vi "r3_Pick&Place_module_sensor_glueDespRev.vi"() -> ()   [LabVIEW 2016]
uses:
  Classes/Controllers/I-O/Copy of NI-DAQ Folder/NI-DAQ.lvclass
  D:/INTT/V1/Classes/Controllers/I-O/Copy of I-O Folder/I-O.lvclass
  Classes/Controllers/Dispenser/Copy of Ultimus V2 Folder/Ultimus V2.lvclass
  <vilib>/Analysis/coordinate.llb/2D Cartesian Coordinate Rotation (Scalar).vi
  <vilib>/Utility/file.llb/Read Delimited Spreadsheet (DBL).vi
  <vilib>/Utility/file.llb/Write Delimited Spreadsheet (DBL).vi
  Classes/Controllers/Motion/Copy of Motion Folder/Motion.lvclass
  Classes/Controllers/Camera/Copy of Controller Folder/Controller.lvclass
  <vilib>/Analysis/NI_AALPro.lvlib
  Classes/Controllers/I-O/Copy of I-O Folder/I-O.lvclass
panel:
  in  "sensor pad offset":dbl[][](array[numeric])=[[0.01279, -0.02707, 0.0, 0.0], [0.02738, -0.01377, 0.0, 0.0]]
  out "Sample on HDI aspect to drawing":dbl[][](array[numeric]) format="%#_8g"
  in  "HDI sensor pad positions":dbl[][](array[numeric]) format="%#_12g"
  in  "Values":bool[](array[boolean])=[FALSE, FALSE]
  out "vacuum on?":bool[](array[boolean])
  out "Array 2":dbl[][](array[numeric])
  out "Measured PickupTool position":dbl[][](array[numeric])
  in  "sampel vacuum":i32[](array[numeric])=[15, 19]
  in  "VacChannel for sample":i32=1
  in  "TrayVaccum":bool
  in  "check height? 2":bool
  in  "check height?":bool
  out "Needle parking position":dbl[](array[numeric])
  out "GlueBox":dbl[][](array[numeric])
  out "appended array":dbl[][](array[numeric])
  in  "chip placement height compensation":dbl=-0.47 format="%#_13g"
  out "Sample on HDI":dbl[][](array[numeric]) format="%#_8g"
  in  "Sensor A/B":bool
  out "Gantry current position":dbl[](array[numeric])
  in  "READ Position":bool
  in  "Needle Height Compenstation\n(glue gap)":dbl=0.34
  in  "Needle Alignment":bool
  in  "Parking position":dbl[](array[numeric])=[500.0, 625.0, 0.0, 0.01]
  in  "GOTO":bool
  in  "Default Pickup Tool Position":dbl[][](array[numeric])=[[132.189, 676.043, 47.1693, 0.0326839], [189.108, 526.841, 47.062, 0.0198801]]
  in  "Number of Chips/Sensors \nto be assembled":i32=1
  in  "Default HDI alignment \nmark position":dbl[](array[numeric])=[292.31, 988.829, 78.9737, -0.000591208]
  in  "Default HDI size":dbl[](array[numeric])=[24.3157, 231.332, -0.00999644, -6.1789e-05]
  out "# of tasks excuted":i32
  out "Chips on tray position":dbl[][](array[numeric])
  out "measured HDI size":dbl[](array[numeric])
  in  "Chip tray":dbl[](array[numeric])=[465.031, 710.639, 69.8028, 0.00407755]
  out "Sample position \non HDI":dbl[][](array[numeric]) format="%#_8g"
  in  "Inititalize":bool
  in  "Pick and place":bool
  in  "Deposit Glue":bool
  in  "Measure Pickup Tools":bool
  in  "Measure Samples on tray":bool
  out "default chip and sensor position w.r.t. 1st mark":dbl[][](array[numeric])
  in  "Assembly Type":bool
  in  "Stop":bool
  in  "Measure HDI":bool
  out "Measure HDI top-left":dbl[](array[numeric])
  # "Sensor Tray \nVacuum Channel"
  # "Chips"
  # "Sensor 0.3 -> 200 micron glue thickness\nChips 0.34-> 150 micron glue thickness"
  # "Sensors"
  # "Sensor B short"
  # "Sensors B\n(Short)"
  # "Sensors A\n(Long)"
  # "Chips : -0.47-> 60 micron height gap\n               -0.5 -> 90 micron"
  # "Sensor A long"
  # "ACTIONS"
  # "HDI infomation"
  # "sensor"
  # "chips use channel 0, 2\nsensors use channel 0, 1"
  # "sensor height 69.8471\nchip height 84.693"
  # "Pick and Place"
  # "TYPE A: \nX: 0.01279\nY: -0.02707"
  # "TYPE B: \nX: 0.02738\nY: -0.01377"
  # "type A"
  # "type B"
  # "type A"
  # "type B"
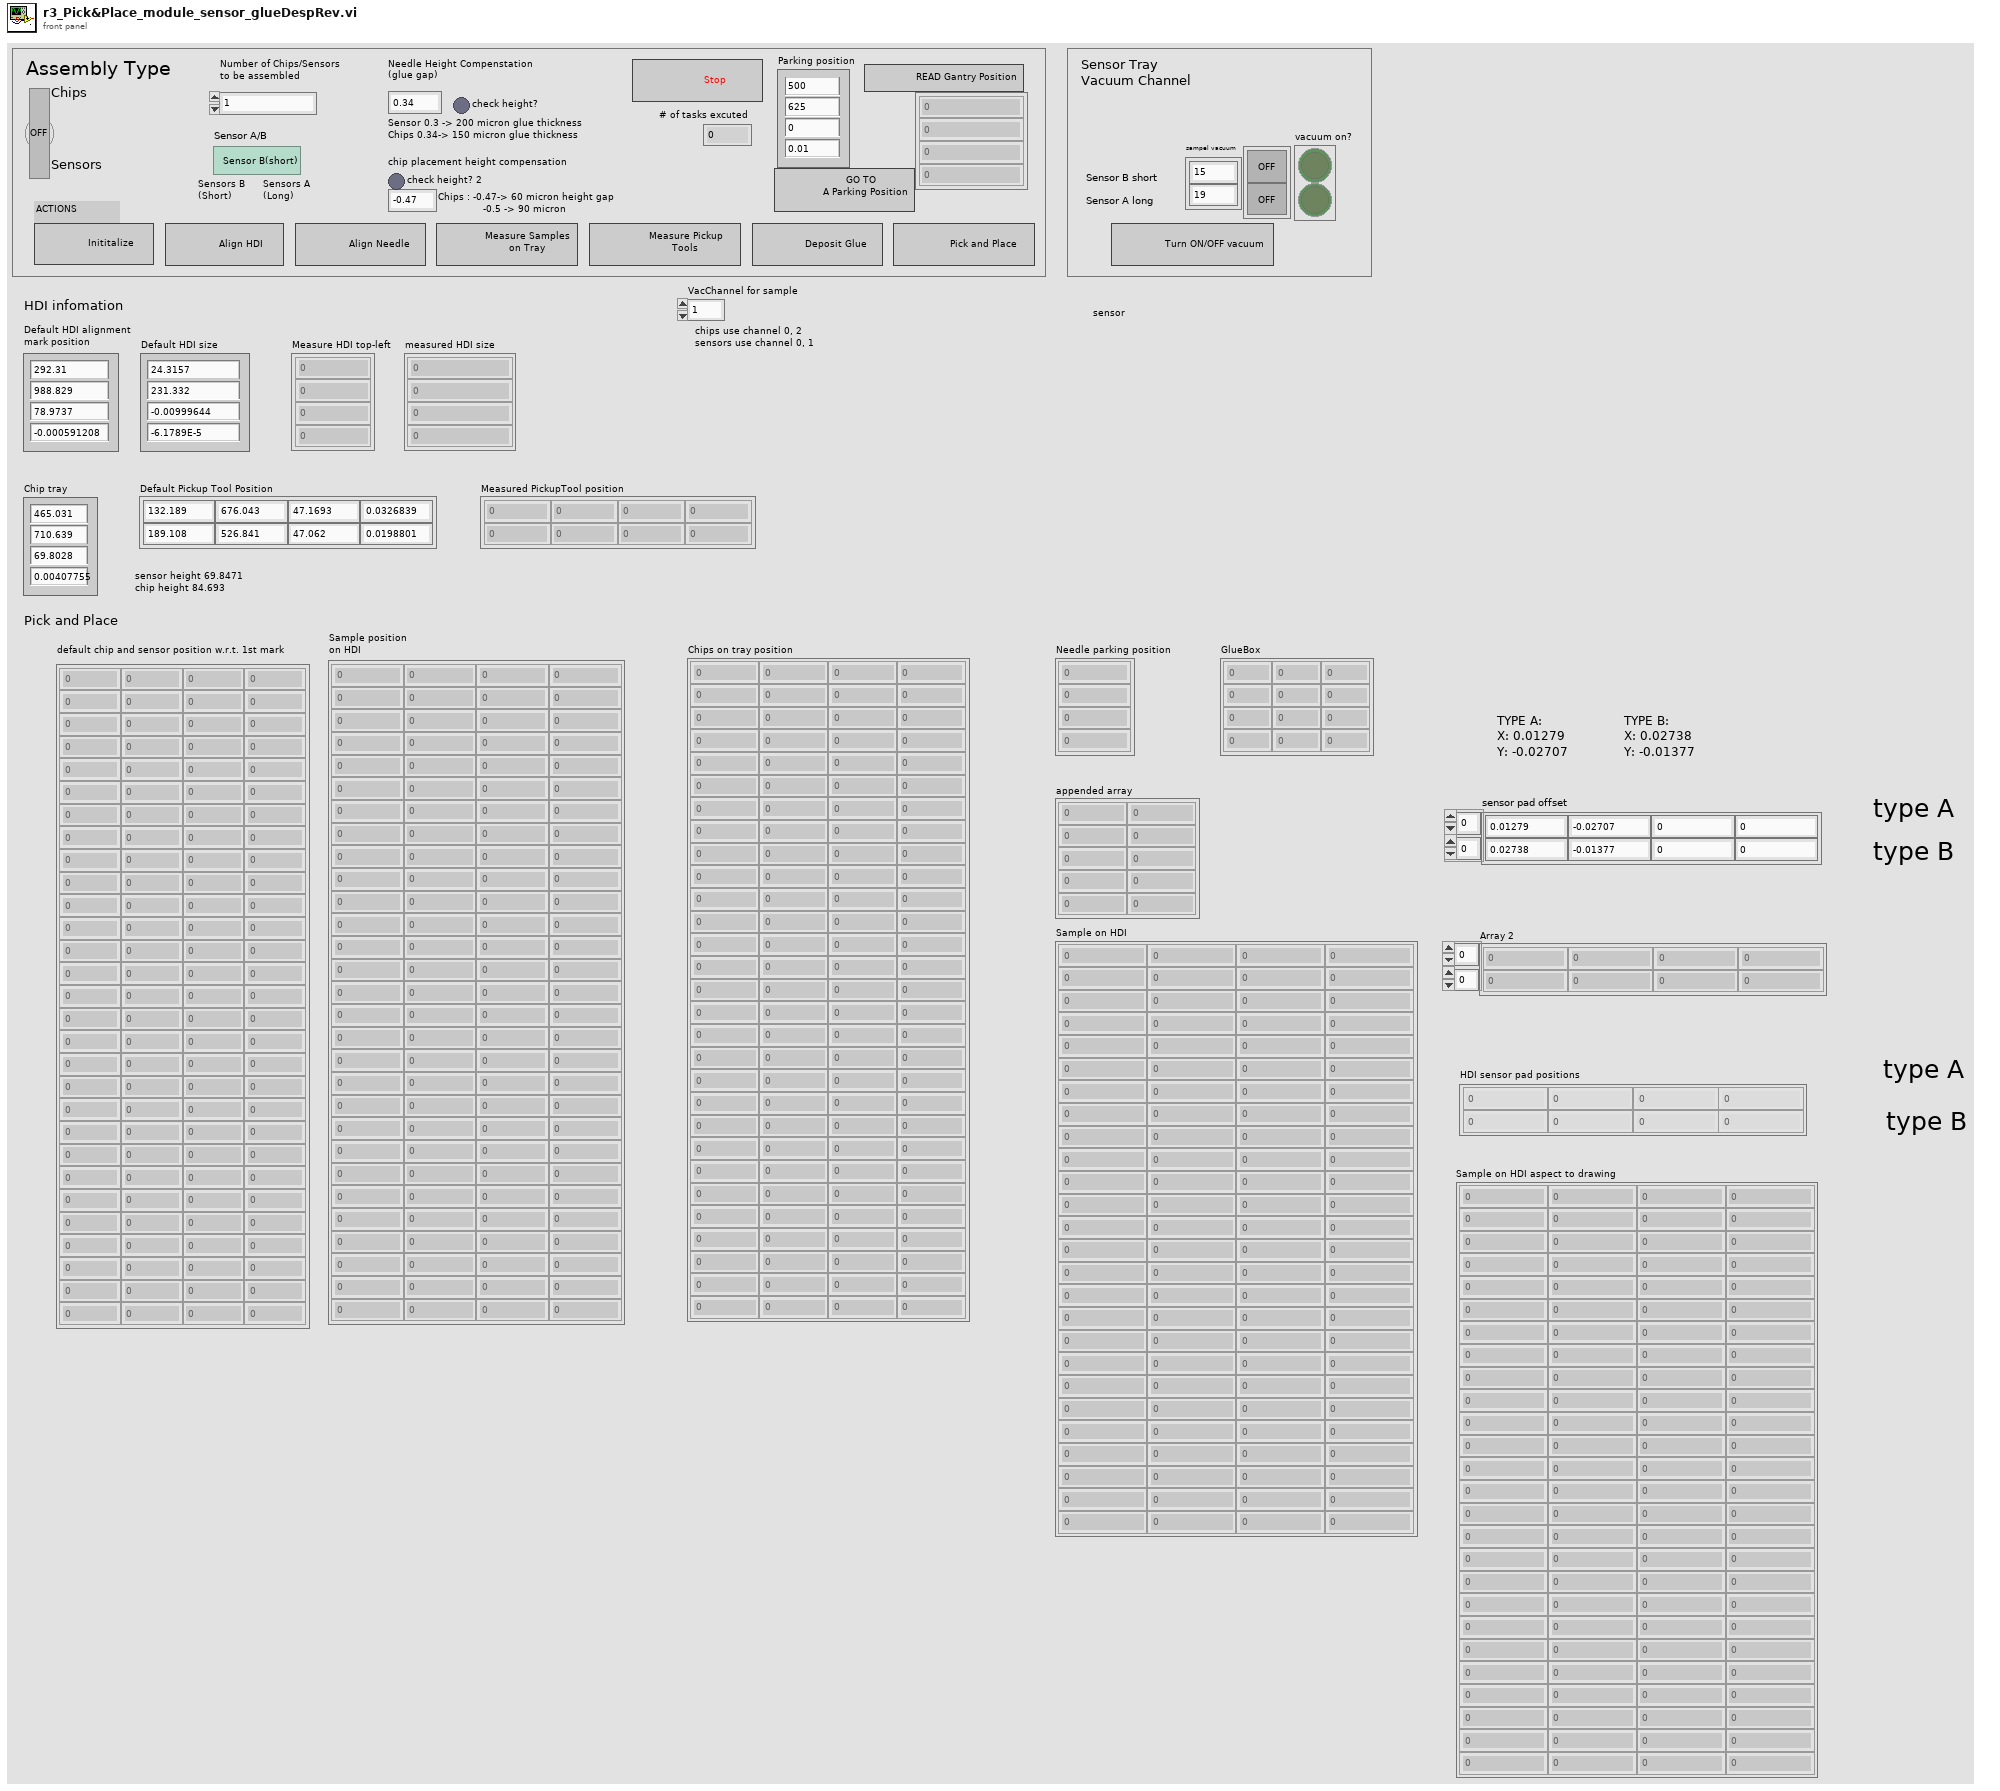
[diagram p1: front panel]
types:
  T1 = typedef "Controller.lvclass/Controllers.ctl" = cluster{"Copy of Motion.lvclass":refnum<class "Motion.lvclass">, "Copy of I-O.lvclass":refnum<class "I-O.lvclass">, "Copy of Dispenser.lvclass":refnum<class "Dispenser.lvclass">}
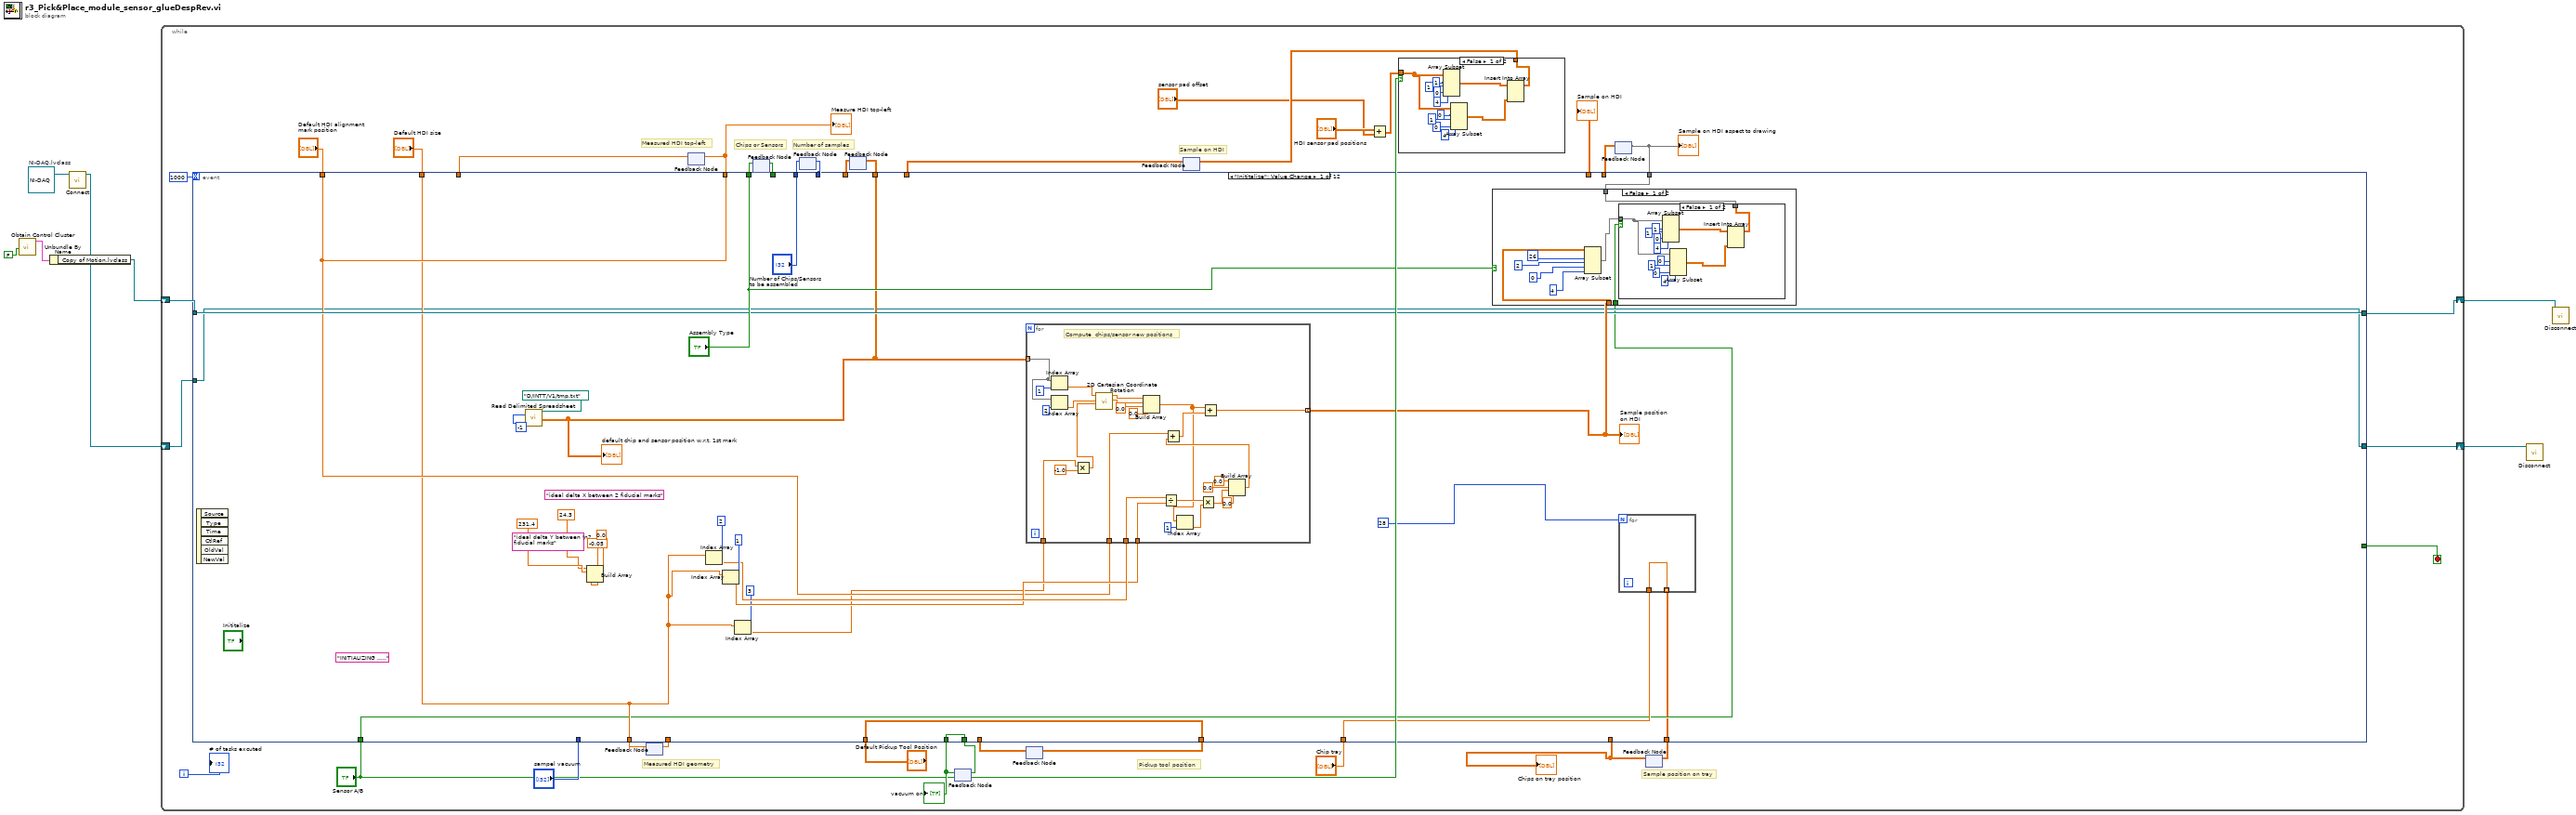
[diagram p0: block diagram]
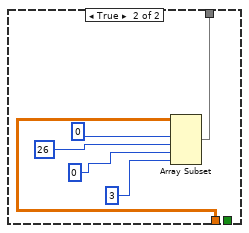
[diagram p4: hidden frame]
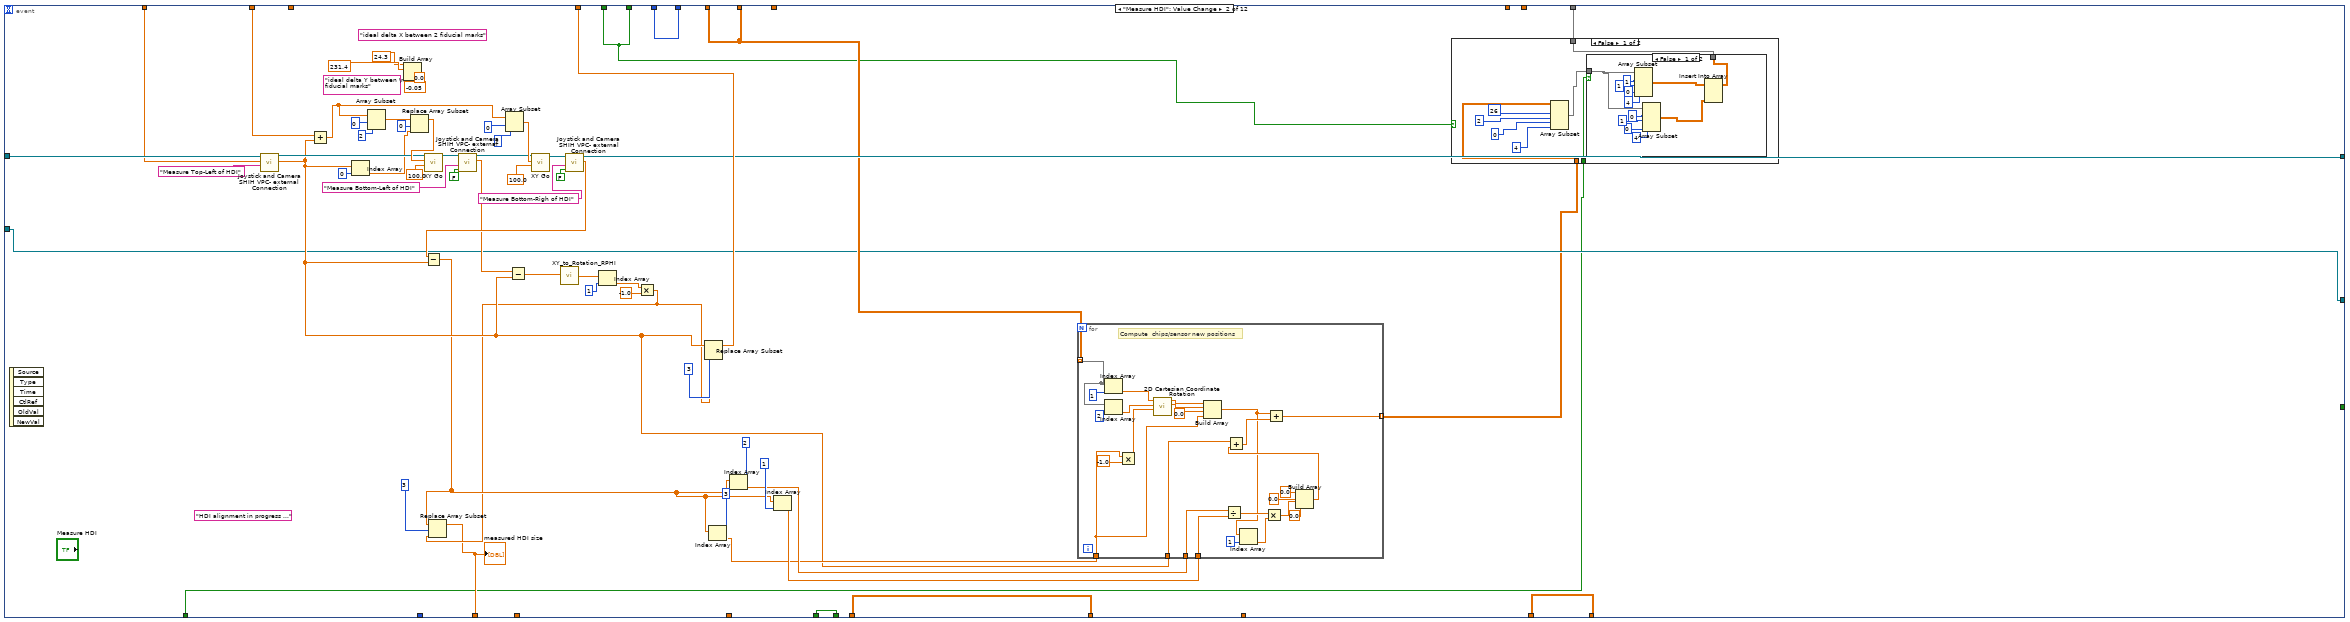
[diagram p5: hidden frame]
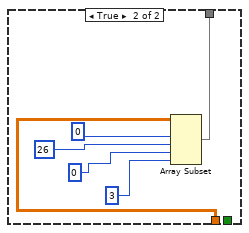
[diagram p7: hidden frame]
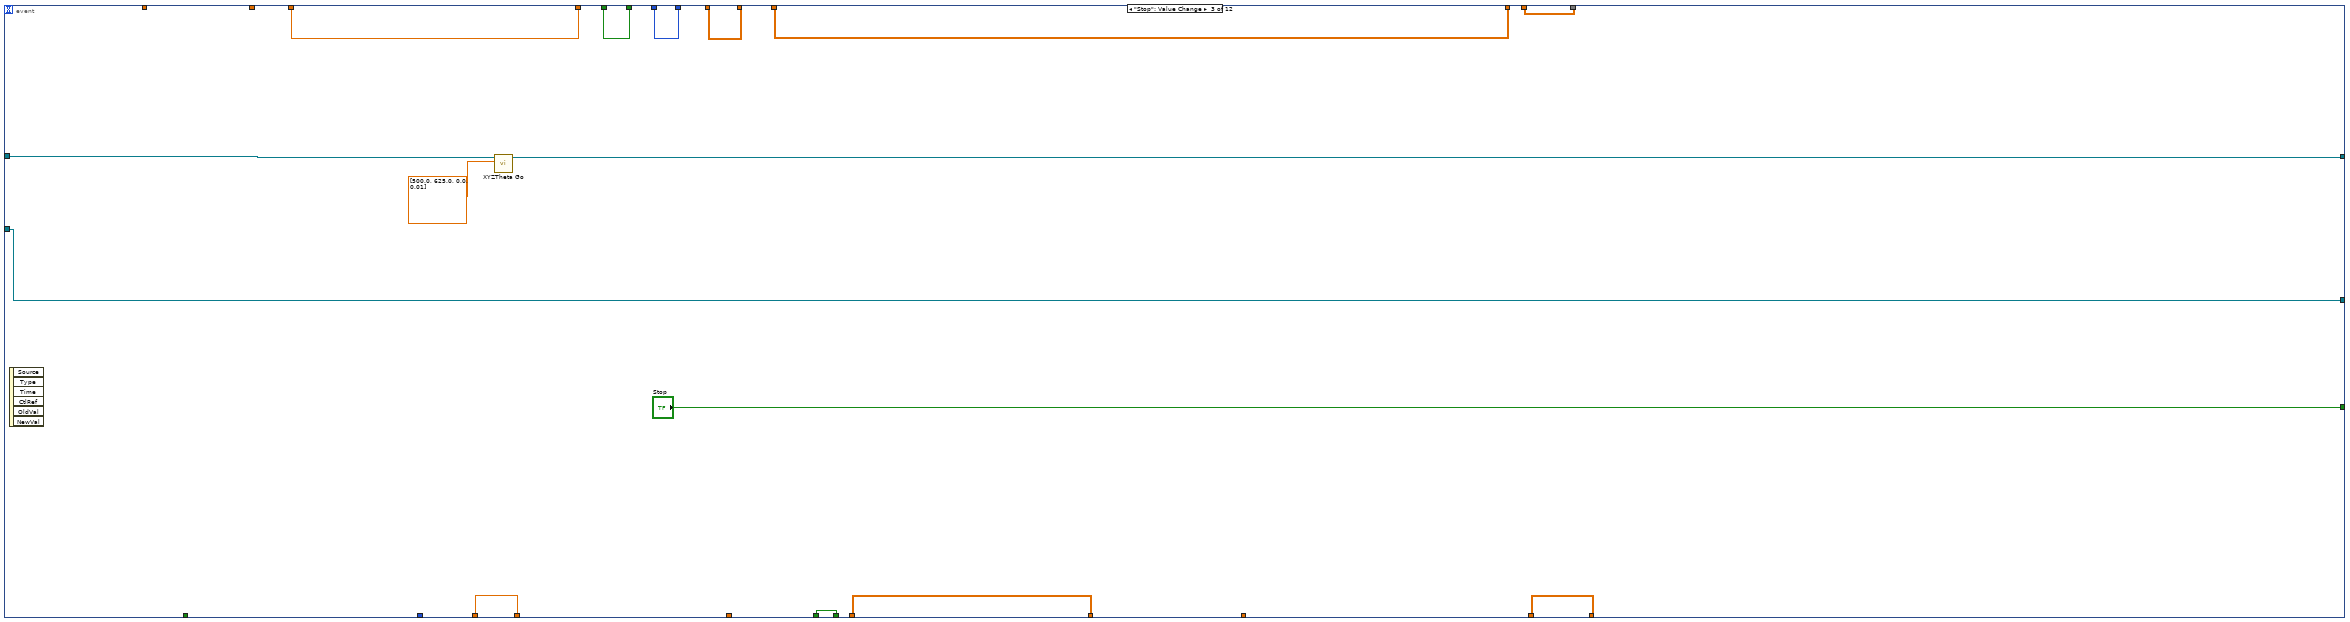
[diagram p8: hidden frame]
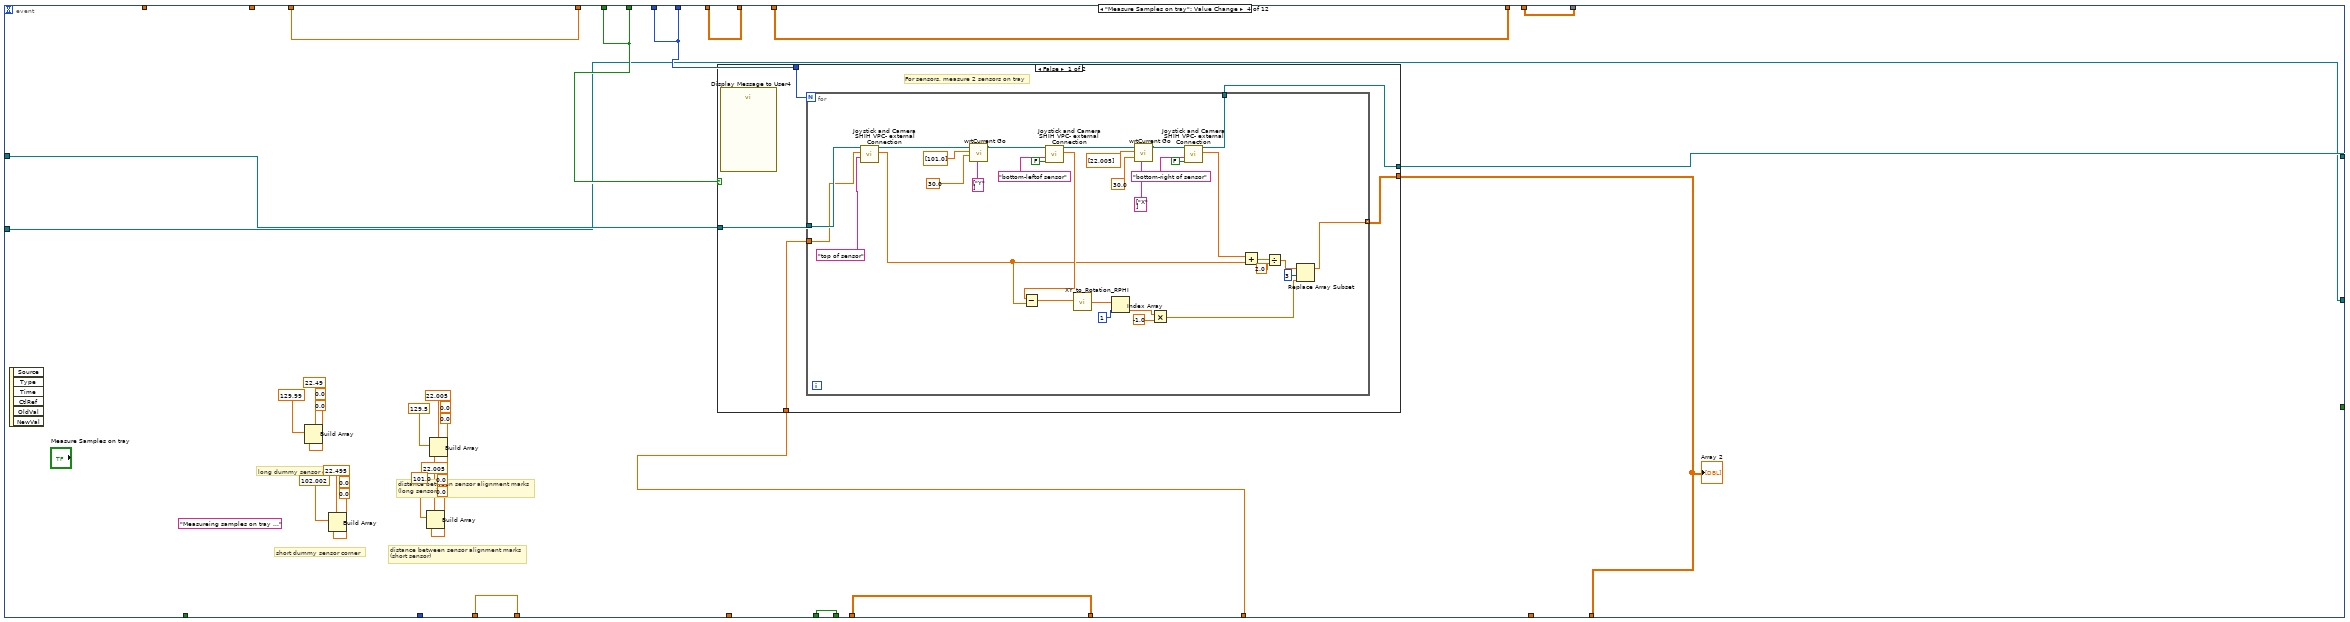
[diagram p9: hidden frame]
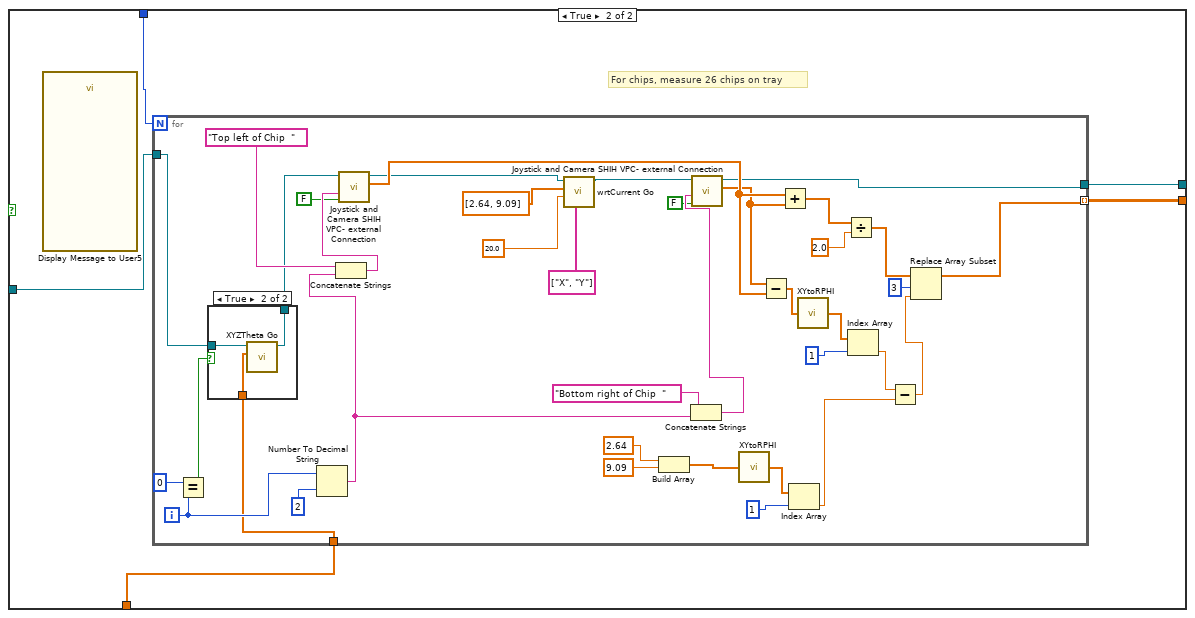
[diagram p10: hidden frame]
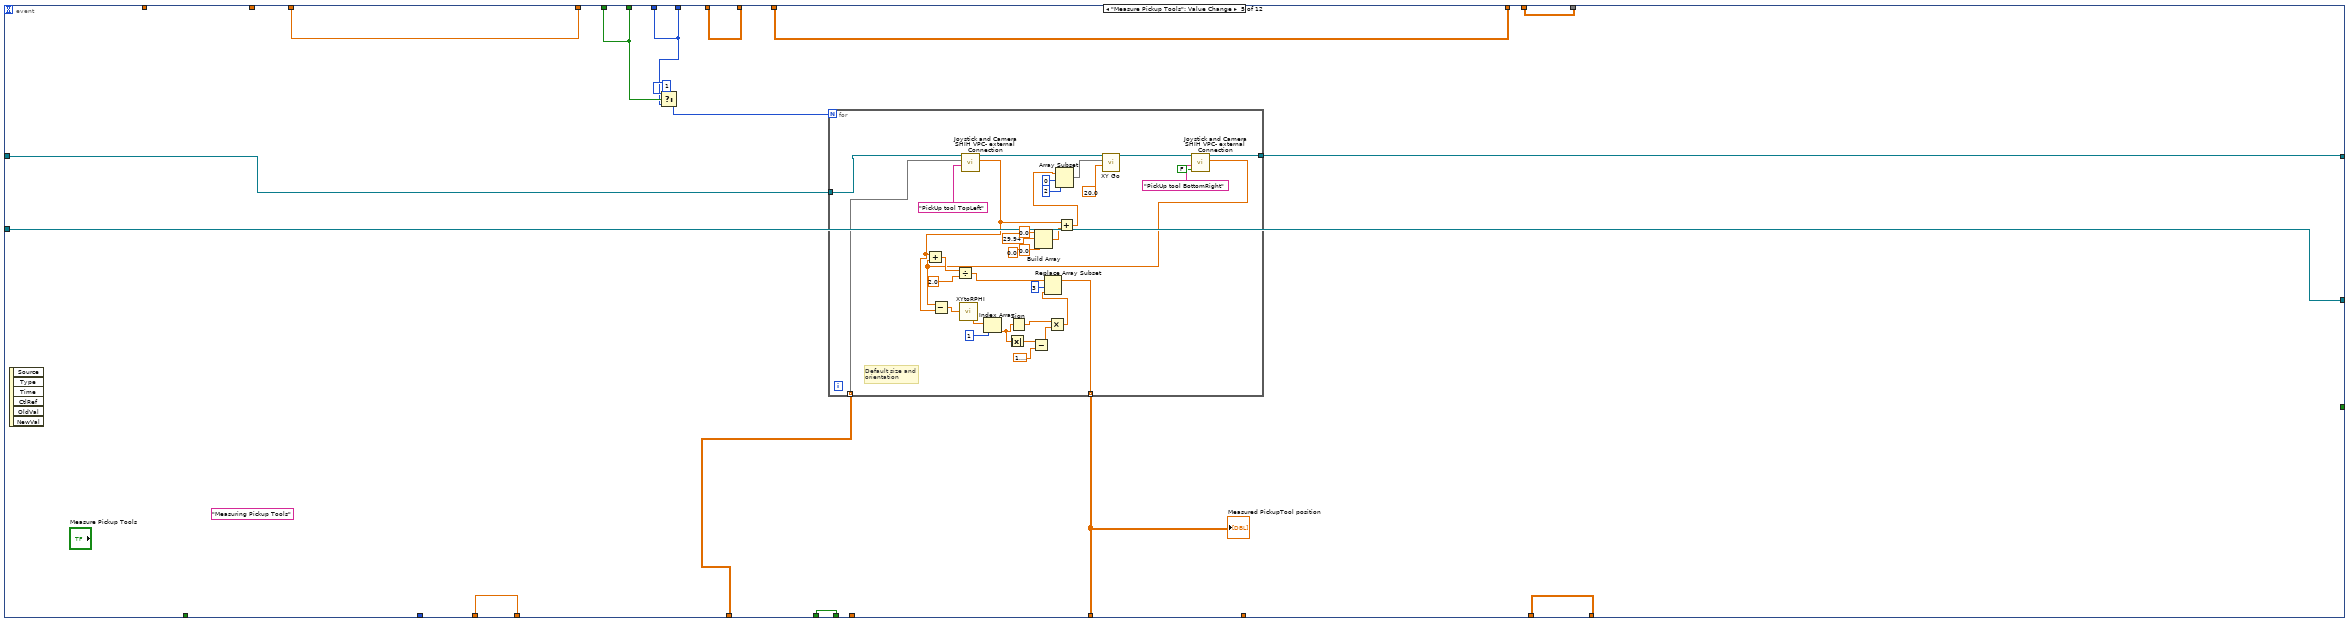
[diagram p12: hidden frame]
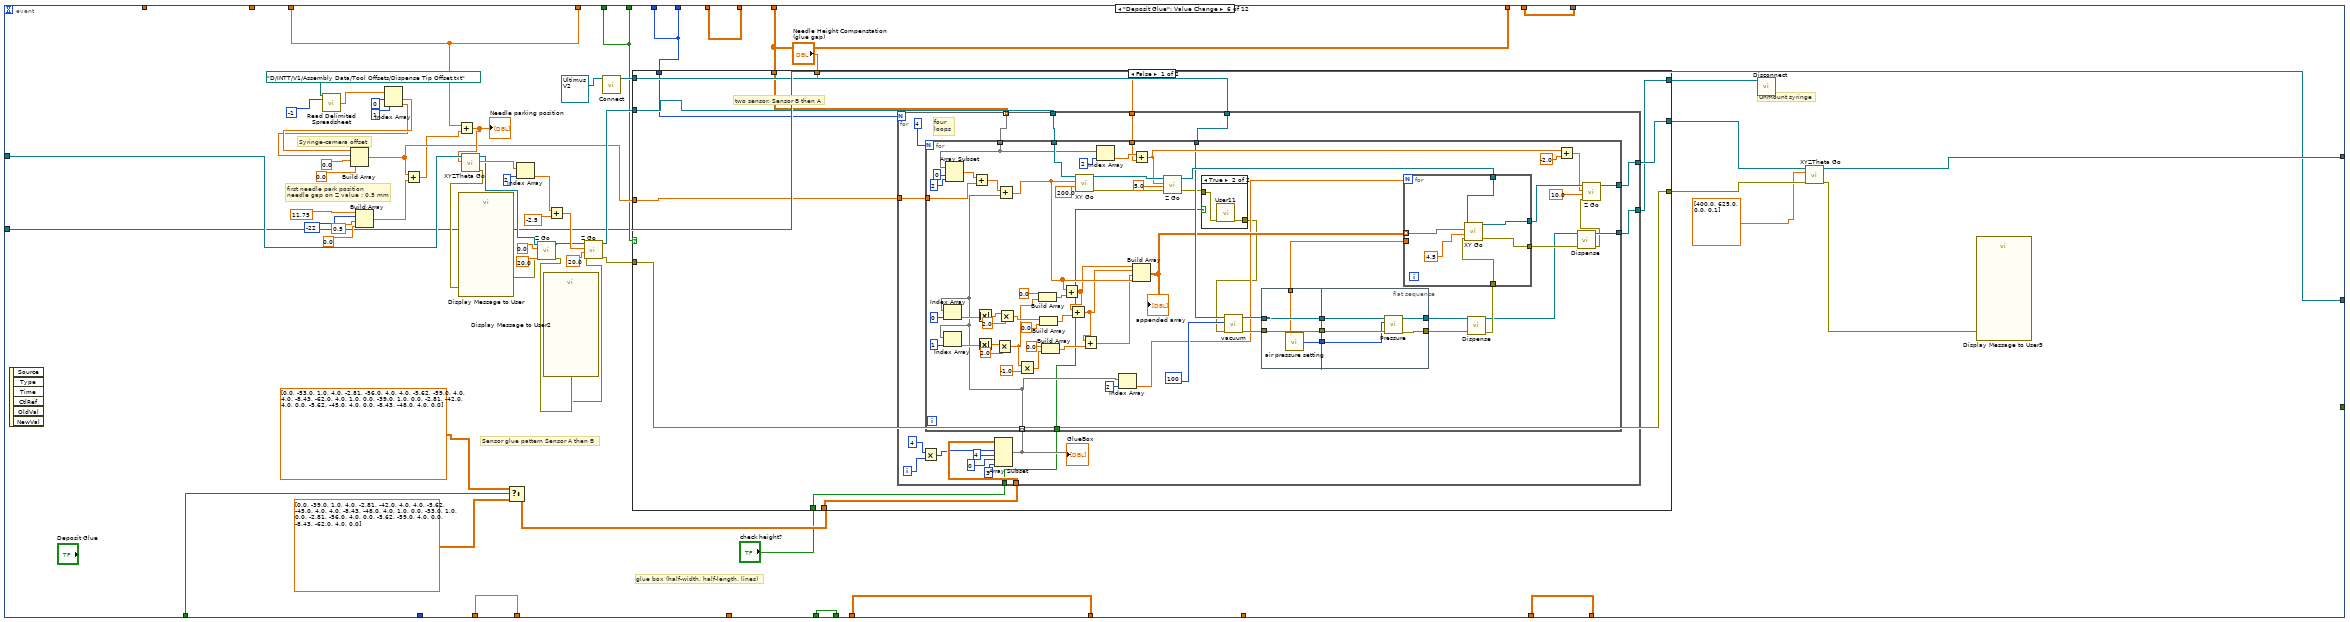
[diagram p13: hidden frame]
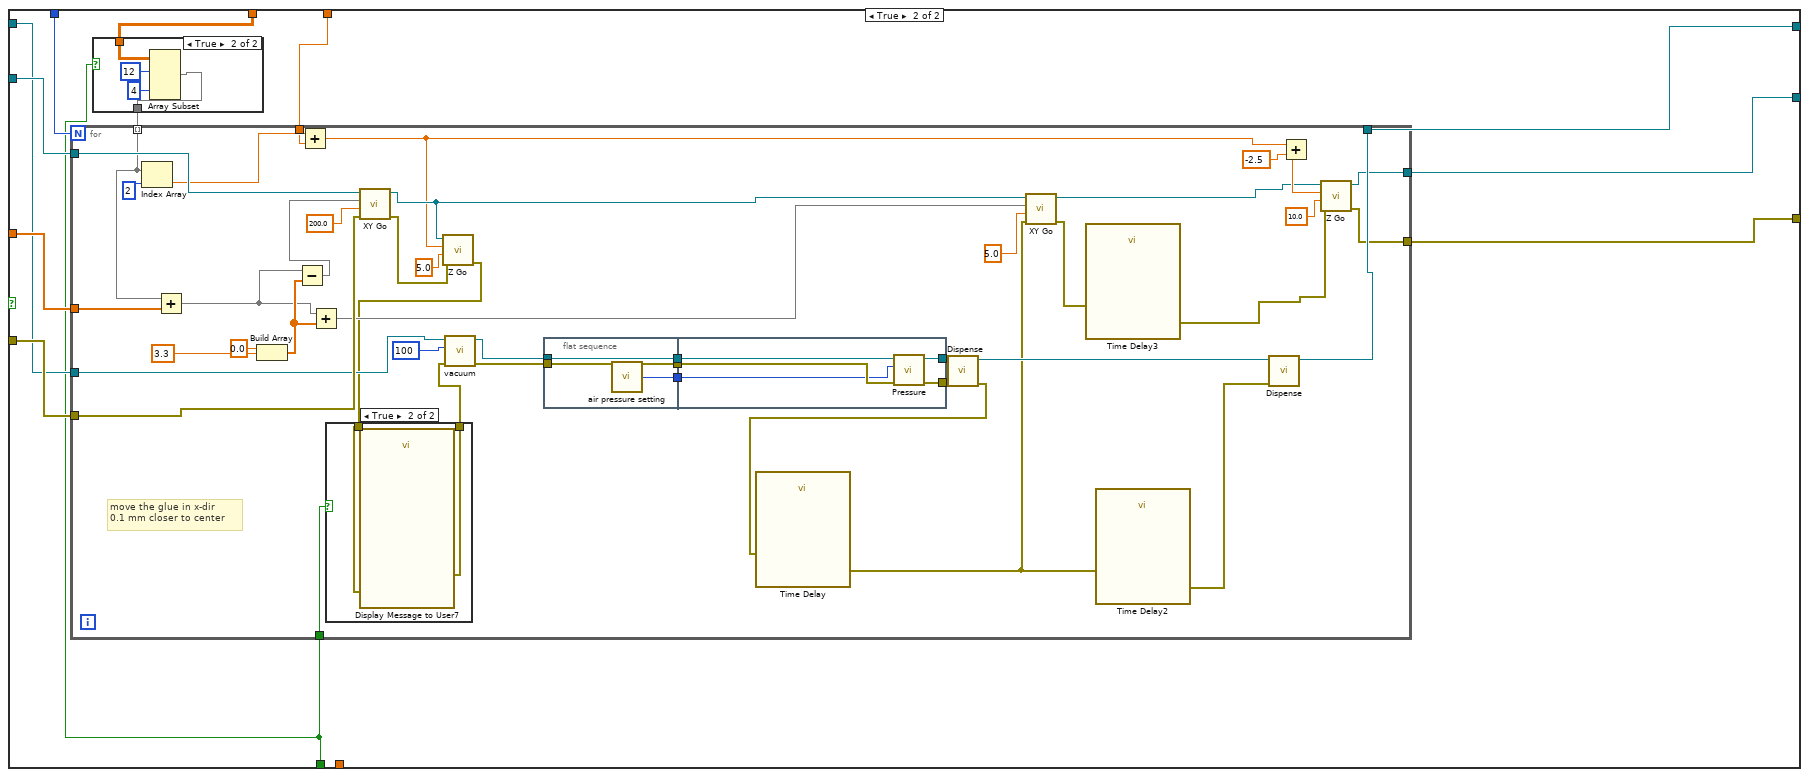
[diagram p15: hidden frame]
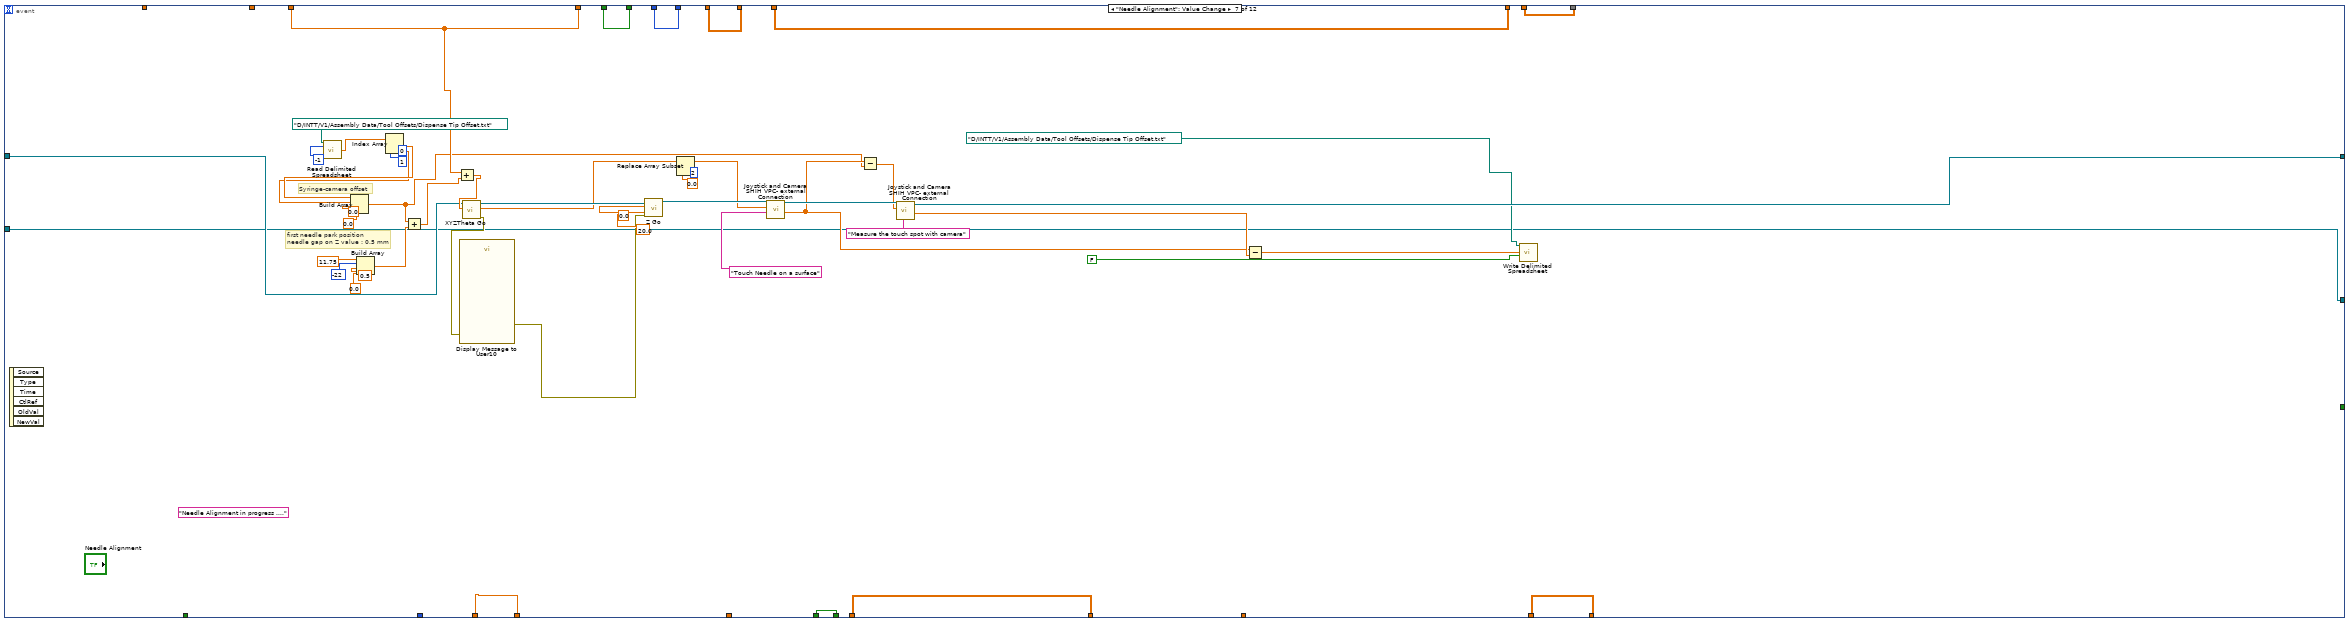
[diagram p18: hidden frame]
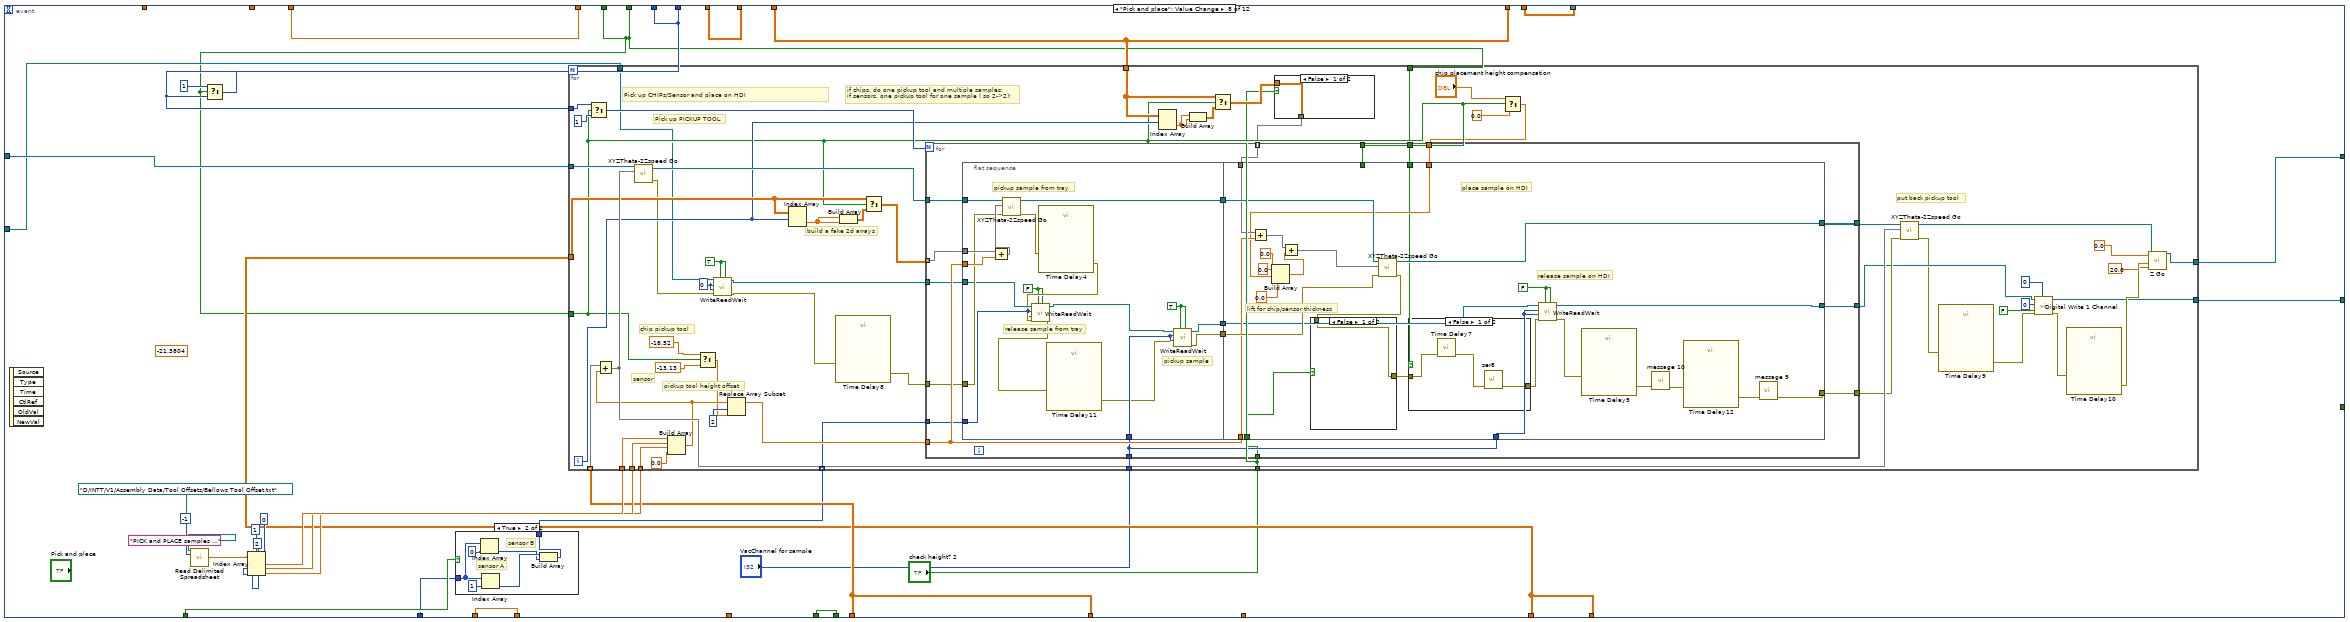
[diagram p19: hidden frame]
diagram:
  w3 = refnum<class "NI-DAQ.lvclass"> refnum  # NI-DAQ.lvclass
  n1 = call "Obtain Control Cluster.vi"("I/O"=FALSE) -> ("Control Out"=w7:T1)  [unwired: 10 in]
  n2 = Unbundle By Name(w7) -> ("Copy of Motion.lvclass"=w5:refnum<class "Motion.lvclass">)
  n3 = call-dynamic "Connect.vi"("NI-DAQ in"=w3) -> ("NI-DAQ out"=w2:refnum<class "NI-DAQ.lvclass">)  [unwired: 9 in, 1 out]
  n4 = while {
    shift-right: [w32] -> w4
    shift-left: w5 -> [w44]
    shift-right: [w20] -> w1
    shift-left: w2 -> [w21]
    i -> [w31]
    stop <- w43 stop-if-true
    # "Pickup tool position"
    # "Chips or Sensors"
    # "Number of samples"
    # "Measured HDI geometry"
    # "Sample position on tray"
    # "Measured HDI top-left"
    # "Sample on HDI"
    n5 = feedback #1() -> (w39:dbl[])  [unwired: 1 in]
    n6 = feedback #2() -> (w41:dbl[])  [unwired: 1 in]
    n7 = feedback #3() -> (w36:bool)  [unwired: 1 in]
    n8 = feedback #4() -> (w30:i32)  [unwired: 1 in]
    n9 = feedback #5() -> (w25:dbl[][])  [unwired: 1 in]
    n10 = feedback #6() -> (w17:bool[])  [unwired: 1 in]
    n11 = feedback #7() -> (w33:dbl[][])  [unwired: 1 in]
    n12 = feedback #8() -> (w38:dbl[][])  [unwired: 1 in]
    n13 = Add(x="HDI sensor pad positions", y="sensor pad offset") -> (x+y=w9:dbl[][])
    n14 = case shown="False" "Sensor A/B" {
      tunnel: w9 -> [w48 w57]
      tunnel: [w45 w57] -> w15
      frame False {
        n15 = Array Subset(array=w48, index (row)=1 ("index"), length (row)=1 ("length"), index (col)=0 ("index"), length (col)=4 ("length")) -> (w47:dbl[][])
        n16 = Array Subset(array=w48, index (row)=0 ("index"), length (row)=1 ("length"), index (col)=0 ("index"), length (col)=4 ("length")) -> (w46:dbl[][])
        n17 = Insert Into Array(array=w47, new element=w46) -> (w45:dbl[][])  [unwired: 2 in]
      }
      frame True {
      }
    }
    n18 = feedback-in #8(w15) -> ()
    n19 = feedback #9() -> (w12:dbl[][])  [unwired: 1 in]
    n20 = feedback #10() -> (w22:dbl[][])  [unwired: 1 in]
    "Chips on tray position" <- w22
    n21 = event shown="[0] \"Inititalize\": Value Change" {
      selector: _ -> [_ _ _ _ _ _ _ _ _ _ _ _]
      dyn-events: _ -> [_ _ _ _ _ _ _ _ _ _ _ _]
      timeout: 1000 -> [_ _ _ _ _ _ _ _ _ _ _ _]
      tunnel: w44 -> [w71 w198 w265 w295 w394 w463 w691 w748 w894 w917 w942 w946]
      tunnel: [_ _ "Stop" _ _ _ _ _ _ _ _ _] -> w43
      tunnel: [w68 w195 w258 w289 w385 w444 w699 w732 w903 w911 w938 w956] -> w42
      tunnel: w41 -> [_ _ w258 w289 w385 w444 w699 w732 w903 w911 w938 w956]
      tunnel: ["Assembly Type" w142 w262 w293 w390 w447 w698 w722 w902 w912 w939 w955] -> w37
      tunnel: [w64 w145 w257 w288 w384 w440 w694 w731 w898 w910 w937 w950] -> w40
      tunnel: w39 -> [_ _ w257 w288 w384 w440 w694 w731 w898 w910 w937 w950]
      tunnel: [_ _ w259 w290 w387 w446 w695 w737 w899 w915 w941 w944] -> w14
      tunnel: w38 -> [_ _ w259 w290 w387 w446 w695 w737 w899 w915 w941 w944]
      tunnel: w36 -> [_ w142 w262 w293 w390 w447 w698 w722 w902 w912 w939 w955]
      tunnel: w30 -> [_ w186 w261 w292 w389 w445 w697 w734 w901 w913 w934 w954]
      tunnel: [w58 w184 w255 w269 w383 w442 w692 w735 w896 w908 w935 w952] -> w35
      tunnel: w22 -> [_ w184 w255 _ w383 w442 w692 w735 w896 w908 w935 w952]
      tunnel: [w67 w185 w256 w287 w393 w441 w693 w736 w897 w909 w936 w951] -> w34
      tunnel: w33 -> [_ w185 w256 w287 _ w441 w693 w736 w897 w909 w936 w951]
      tunnel: [w71 w194 w263 w294 w392 w448 w683 w738 w893 w916 w942 w946] -> w32
      tunnel: ["Number of Chips/Sensors \nto be assembled" w186 w261 w292 w389 w445 w697 w734 w901 w913 w934 w954] -> w29
      tunnel: "Default HDI alignment \nmark position" -> [w68 w193 _ _ _ _ _ _ _ _ _ _]
      tunnel: "Default HDI size" -> [w64 w192 _ _ _ _ _ _ _ _ _ _]
      tunnel: [w69 w187 w260 w291 w386 w439 w696 w733 w900 w914 w940 w953] -> w26
      tunnel: w25 -> [_ w187 w260 w291 w386 w439 w696 w733 w900 w914 w940 w953]
      tunnel: "Default Pickup Tool Position" -> [w67 _ _ _ w388 _ _ _ _ _ _ _]
      tunnel: "Chip tray" -> [w66 _ _ w286 _ _ _ _ _ _ _ _]
      tunnel: "Sensor A/B" -> [w61 w139 _ _ _ w438 _ w730 _ _ _ _]
      tunnel: w21 -> [w62 w144 w253 w268 w382 w433 w674 w727 w895 w906 w933 w947]
      tunnel: [w62 w144 w253 w268 w382 w433 w674 w728 w895 w906 w919 w945] -> w20
      tunnel: "sampel vacuum" -> [_ _ _ _ _ _ _ w724 _ _ w921 w948]
      tunnel: [w60 w143 w252 w267 w381 w432 w673 w723 w891 w905 w920 w949] -> w18
      tunnel: w17 -> [w60 w143 w252 w267 w381 w432 w673 w723 w891 w905 w920 _]
      tunnel: [w59 w140 w251 w266 w380 w431 w672 w721 w890 w904 w918 w943] -> w13
      tunnel: w12 -> [_ _ w251 w266 w380 w431 w672 w721 w890 w904 w918 w943]
      event "Inititalize": Value Change {
        (unwired) "INITIALIZING ....." ("String")
        (unwired) "ideal delta Y between \n2 fiducial marks"
        (unwired) "ideal delta X between 2 fiducial marks"
        n22 = event-data() -> ()  [unwired: 1 in, 6 out]
        n23 = call-poly <vilib>:"Read Delimited Spreadsheet.vi"("file path (dialog if empty)"=path "D:/INTT/V1/tmp.txt", "number of rows (all:-1)"=-1) -> ("all rows"=w69:dbl[][])  [unwired: 8 in, 5 out]
        "default chip and sensor position w.r.t. 1st mark" <- w69
        n24 = Build Array(24.3 ("y"), 231.4 ("y"), 0.0 ("element"), -0.05 ("element")) -> ()  [unwired: 1 out]
        n25 = Index Array(array=w64, index=2) -> (element=w80:dbl)
        n26 = Index Array(array=w64, index=1) -> (element=w79:dbl)
        n27 = Index Array(array=w64, index=3) -> (element=w63:dbl)
        n28 = for {
          tunnel: w69 -> [w131] mode=indexing
          tunnel: w63 -> [w114]
          tunnel: w68 -> [w123]
          tunnel: [w130] -> w73 mode=indexing
          tunnel: w80 -> [w129]
          tunnel: w79 -> [w120]
          # "Compute  chips/sensor new positions"
          n29 = Index Array(array=w131, index=1) -> (element=w135:dbl)
          n30 = Index Array(array=w131, index=2) -> (element=w134:dbl)
          n31 = Multiply(x=w114, y=-1.0) -> (x*y=w115:dbl)
          n32 = call-poly <vilib>:"2D Cartesian Coordinate Rotation.vi"("theta"=w115, "y"=w134, "x"=w135) -> ("y out"=w137:dbl, "x out"=w136:dbl)  [unwired: 6 in, 1 out]
          n33 = Build Array(w136, w137, 0.0 ("element"), 0.0 ("element")) -> (w117:dbl[])
          n34 = Divide(x=w129, y=w120) -> (x/y=w128:dbl)
          n35 = Index Array(array=w117, index=1) -> (element=w118:dbl)
          n36 = Multiply(x=w128, y=w118) -> (x*y=w124:dbl)
          n37 = Build Array(0.0 ("element"), 0.0 ("element"), w124, 0.0 ("element")) -> (w122:dbl[])
          n38 = Add(x=w123, y=w122) -> (x+y=w121:dbl[])
          n39 = Add(x=w117, y=w121) -> (x+y=w130:dbl[])
        }
        "Sample position \non HDI" <- w73
        n40 = case shown="False" "Assembly Type" {
          tunnel: w73 -> [w88 w108]
          tunnel: [w86 w106] -> w59
          tunnel: w61 -> [w85 _]
          frame False {
            n41 = Array Subset(array=w88, index (row)=26 ("index"), length (row)=2 ("length"), index (col)=0, length (col)=4 ("length")) -> (w87:dbl[][])
            n42 = case shown="False" w85 {
              tunnel: w87 -> [w96 w105]
              tunnel: [w93 w105] -> w86
              frame False {
                n43 = Array Subset(array=w96, index (row)=1 ("index"), length (row)=1 ("length"), index (col)=0 ("index"), length (col)=4 ("length")) -> (w95:dbl[][])
                n44 = Array Subset(array=w96, index (row)=0 ("index"), length (row)=1 ("length"), index (col)=0 ("index"), length (col)=4 ("length")) -> (w94:dbl[][])
                n45 = Insert Into Array(array=w95, new element=w94) -> (w93:dbl[][])  [unwired: 2 in]
              }
              frame True {
              }
            }
          }
          frame True {
            n46 = Array Subset(array=w108, index (row)=0 ("index"), length (row)=26 ("length"), index (col)=0, length (col)=3 ("length")) -> (w106:dbl[][])
          }
        }
        n47 = for {
          N: 28 -> [_]
          tunnel: w66 -> [w112]
          tunnel: [w112] -> w58 mode=indexing
        }
      }
      event "Measure HDI": Value Change {
        (unwired) "ideal delta Y between \n2 fiducial marks"
        (unwired) "ideal delta X between 2 fiducial marks"
        (unwired) "HDI alignment in progress ..." ("String")
        n48 = event-data() -> ()  [unwired: 1 in, 6 out]
        n49 = call "Joystick and Camera SHIH VPC- external Connection.vi"("Motion in"=w198, "XYZTheta"=w193, "Measurement Point"="Measure Top-Left of HDI") -> ("Motion out"=w162:refnum<class "Motion.lvclass">, "Sum"=w151:dbl[])  [unwired: 4 in, 2 out]
        n50 = Add(x=w192, y=w151) -> (x+y=w166:dbl[])
        n51 = Index Array(array=w151, index=0) -> (element=w153:dbl)
        n52 = Array Subset(array=w166, index=0, length=2) -> (w165:dbl[])
        n53 = Build Array(24.3 ("y"), 231.4 ("y"), 0.0 ("element"), -0.05 ("element")) -> ()  [unwired: 1 out]
        n54 = Replace Array Subset(array=w165, new element=w153, index=0) -> (w163:dbl[])
        n55 = call-dynamic "XY Go.vi"("Speed"=100.0, "XY"=w163, "Motion in"=w162) -> ("Motion out"=w170:refnum<class "Motion.lvclass">)  [unwired: 7 in, 1 out]
        n56 = call "Joystick and Camera SHIH VPC- external Connection.vi"("Motion in"=w170, "Measurement Point"="Measure Bottom-Left of HDI", "Inital GO"=FALSE) -> ("Motion out"=w161:refnum<class "Motion.lvclass">, "Sum"=w152:dbl[])  [unwired: 4 in, 2 out]
        n57 = Array Subset(array=w166, index=0, length=2) -> (w176:dbl[])
        n58 = Subtract(x=w152, y=w151) -> (x-y=w160:dbl[])
        n59 = call-dynamic "XY Go.vi"("Speed"=100.0, "XY"=w176, "Motion in"=w161) -> ("Motion out"=w180:refnum<class "Motion.lvclass">)  [unwired: 7 in, 1 out]
        n60 = call "XY_to_Rotation_RPHI.vi"("X-Y"=w160) -> ("r-phi"=w156:dbl[])
        n61 = call "Joystick and Camera SHIH VPC- external Connection.vi"("Motion in"=w180, "Measurement Point"="Measure Bottom-Righ of HDI", "Inital GO"=FALSE) -> ("Motion out"=w194:refnum<class "Motion.lvclass">, "Sum"=w197:dbl[])  [unwired: 4 in, 2 out]
        n62 = Subtract(x=w197, y=w151) -> (x-y=w148:dbl[])
        n63 = Index Array(array=w156, index=1) -> (element=w149:dbl)
        n64 = Multiply(x=w149, y=-1.0) -> (x*y=w146:dbl)
        n65 = Replace Array Subset(array=w148, new element=w146, index=3) -> (w145:dbl[])
        "measured HDI size" <- w145
        n66 = Replace Array Subset(array=w151, new element=w146, index=3) -> (w195:dbl[])
        n67 = Index Array(array=w148, index=3) -> (element=w182:dbl)
        n68 = Index Array(array=w148, index=2) -> (element=w189:dbl)
        n69 = Index Array(array=w148, index=1) -> (element=w188:dbl)
        n70 = for {
          tunnel: w187 -> [w243] mode=indexing
          tunnel: w182 -> [w227]
          tunnel: w151 -> [w235]
          tunnel: [w242] -> w141 mode=indexing
          tunnel: w189 -> [w241]
          tunnel: w188 -> [w232]
          # "Compute  chips/sensor new positions"
          n71 = Index Array(array=w243, index=1) -> (element=w247:dbl)
          n72 = Index Array(array=w243, index=2) -> (element=w246:dbl)
          n73 = Multiply(x=w227, y=-1.0) -> (x*y=w226:dbl)
          n74 = call-poly <vilib>:"2D Cartesian Coordinate Rotation.vi"("theta"=w226, "y"=w246, "x"=w247) -> ("y out"=w249:dbl, "x out"=w248:dbl)  [unwired: 6 in, 1 out]
          n75 = Build Array(w248, w249, 0.0 ("element"), w227) -> (w229:dbl[])
          n76 = Divide(x=w241, y=w232) -> (x/y=w240:dbl)
          n77 = Index Array(array=w229, index=1) -> (element=w230:dbl)
          n78 = Multiply(x=w240, y=w230) -> (x*y=w236:dbl)
          n79 = Build Array(0.0 ("element"), 0.0 ("element"), w236, 0.0 ("element")) -> (w234:dbl[])
          n80 = Add(x=w235, y=w234) -> (x+y=w233:dbl[])
          n81 = Add(x=w229, y=w233) -> (x+y=w242:dbl[])
        }
        n82 = case shown="False" w142 {
          tunnel: w141 -> [w202 w222]
          tunnel: [w200 w220] -> w140
          tunnel: w139 -> [w199 _]
          frame False {
            n83 = Array Subset(array=w202, index (row)=26 ("index"), length (row)=2 ("length"), index (col)=0, length (col)=4 ("length")) -> (w201:dbl[][])
            n84 = case shown="False" w199 {
              tunnel: w201 -> [w210 w219]
              tunnel: [w207 w219] -> w200
              frame False {
                n85 = Array Subset(array=w210, index (row)=1 ("index"), length (row)=1 ("length"), index (col)=0 ("index"), length (col)=4 ("length")) -> (w209:dbl[][])
                n86 = Array Subset(array=w210, index (row)=0 ("index"), length (row)=1 ("length"), index (col)=0 ("index"), length (col)=4 ("length")) -> (w208:dbl[][])
                n87 = Insert Into Array(array=w209, new element=w208) -> (w207:dbl[][])  [unwired: 2 in]
              }
              frame True {
              }
            }
          }
          frame True {
            n88 = Array Subset(array=w222, index (row)=0 ("index"), length (row)=26 ("length"), index (col)=0, length (col)=3 ("length")) -> (w220:dbl[][])
          }
        }
      }
      event "Stop": Value Change {
        n89 = event-data() -> ()  [unwired: 1 in, 6 out]
        n90 = call "XYZTheta Go.vi"("XYZTheta In"=dbl[] [500.0, 625.0, 0.0, 0.01], "Motion in"=w265) -> ("Motion out"=w263:refnum<class "Motion.lvclass">)  [unwired: 7 in, 2 out]
      }
      event "Measure Samples on tray": Value Change {
        (unwired) "Measureing samples on tray ..." ("String")
        # "long dummy sensor corner"
        # "short dummy sensor corner"
        # "distance between sensor alignment marks\n(short sensor)"
        # "distance between sensor alignment marks\n(long sensor)"
        n91 = event-data() -> ()  [unwired: 1 in, 6 out]
        n92 = Build Array(22.49 ("element"), 129.99 ("element"), 0.0 ("element"), 0.0 ("element")) -> ()  [unwired: 1 out]
        n93 = Build Array(22.495 ("element"), 102.002 ("element"), 0.0 ("element"), 0.0 ("element")) -> ()  [unwired: 1 out]
        n94 = Build Array(22.005 ("element"), 101.0 ("element"), 0.0 ("element"), 0.0 ("element")) -> ()  [unwired: 1 out]
        n95 = Build Array(22.005 ("element"), 129.5 ("element"), 0.0 ("element"), 0.0 ("element")) -> ()  [unwired: 1 out]
        n96 = case shown="False" w293 {
          tunnel: [w297 w337] -> w269
          tunnel: w295 -> [w300 w336]
          tunnel: [w296 w335] -> w294
          tunnel: w292 -> [w299 w334]
          tunnel: w286 -> [w298 w333]
          frame False {
            # "For sensors, measure 2 sensors on tray"
            n97 = call "Display Message to User4"() -> ()  [unwired: 10 in, 2 out]
            n98 = for {
              N: w299 -> [_]
              tunnel: w300 -> [w332]
              tunnel: [w329] -> w296
              tunnel: [w323] -> w297 mode=indexing
              tunnel: w298 -> [w322]
              n99 = call "Joystick and Camera SHIH VPC- external Connection.vi"("Motion in"=w332, "XYZTheta"=w322, "Measurement Point"="top of sensor") -> ("Motion out"=w304:refnum<class "Motion.lvclass">, "Sum"=w311:dbl[])  [unwired: 4 in, 2 out]
              n100 = call-dynamic "wrtCurrent Go.vi"("axis names"=string[] ["Y"], "Speed"=30.0, "distances"=dbl[] [101.0], "Motion in"=w304) -> ("Motion out"=w303:refnum<class "Motion.lvclass">)  [unwired: 6 in, 1 out]
              n101 = call "Joystick and Camera SHIH VPC- external Connection.vi"("Motion in"=w303, "Measurement Point"="bottom-leftof sensor", "Inital GO"=FALSE) -> ("Motion out"=w309:refnum<class "Motion.lvclass">, "Sum"=w313:dbl[])  [unwired: 4 in, 2 out]
              n102 = Subtract(x=w313, y=w311) -> (x-y=w318:dbl[])
              n103 = call "XY_to_Rotation_RPHI.vi"("X-Y"=w318) -> ("r-phi"=w317:dbl[])
              n104 = Index Array(array=w317, index=1) -> (element=w314:dbl)
              n105 = call-dynamic "wrtCurrent Go.vi"("axis names"=string[] ["X"], "Speed"=30.0, "distances"=dbl[] [22.005], "Motion in"=w309) -> ("Motion out"=w310:refnum<class "Motion.lvclass">)  [unwired: 6 in, 1 out]
              n106 = Multiply(x=w314, y=-1.0) -> (x*y=w312:dbl)
              n107 = call "Joystick and Camera SHIH VPC- external Connection.vi"("Motion in"=w310, "Measurement Point"="bottom-right of sensor", "Inital GO"=FALSE) -> ("Motion out"=w329:refnum<class "Motion.lvclass">, "Sum"=w326:dbl[])  [unwired: 4 in, 2 out]
              n108 = Add(x=w326, y=w311) -> (x+y=w327:dbl[])
              n109 = Divide(x=w327, y=2.0) -> (x/y=w325:dbl[])
              n110 = Replace Array Subset(array=w325, new element=w312, index=3) -> (w323:dbl[])
            }
          }
          frame True {
            # "For chips, measure 26 chips on tray"
            n111 = call "Display Message to User5"() -> ()  [unwired: 10 in, 2 out]
            n112 = for {
              N: w334 -> [_]
              tunnel: [w364] -> w337 mode=indexing
              tunnel: w336 -> [w348]
              tunnel: [w344] -> w335
              tunnel: w333 -> [w349]
              i -> [w352]
              n113 = Equal?(x=0, y=w352) -> (x = y?=w350:bool)
              n114 = case shown="True" w350 {
                tunnel: w349 -> [_ w379]
                tunnel: w348 -> [w376 w378]
                tunnel: [w376 w377] -> w347
                frame False {
                }
                frame True {
                  n115 = call "XYZTheta Go.vi"("XYZTheta In"=w379, "Motion in"=w378) -> ("Motion out"=w377:refnum<class "Motion.lvclass">)  [unwired: 7 in, 2 out]
                }
              }
              n116 = Number To Decimal String(number=w352, width (-)=i16 2) -> (decimal integer string=w368:string)
              n117 = Concatenate Strings("Top left of Chip  " ("string"), w368) -> (w362:string)
              n118 = call "Joystick and Camera SHIH VPC- external Connection.vi"("Motion in"=w347, "Measurement Point"=w362, "Inital GO"=FALSE) -> ("Motion out"=w341:refnum<class "Motion.lvclass">, "Sum"=w367:dbl[])  [unwired: 4 in, 2 out]
              n119 = call-dynamic "wrtCurrent Go.vi"("axis names"=string[] ["X", "Y"], "Speed"=20.0, "distances"=dbl[] [2.64, 9.09], "Motion in"=w341) -> ("Motion out"=w342:refnum<class "Motion.lvclass">)  [unwired: 6 in, 1 out]
              n120 = Build Array(2.64 ("element"), 9.09 ("element")) -> (w357:dbl[])
              n121 = Concatenate Strings("Bottom right of Chip  " ("string"), w368) -> (w346:string)
              n122 = call "Joystick and Camera SHIH VPC- external Connection.vi"("Motion in"=w342, "Measurement Point"=w346, "Inital GO"=FALSE) -> ("Motion out"=w344:refnum<class "Motion.lvclass">, "Sum"=w343:dbl[])  [unwired: 4 in, 2 out]
              n123 = call "XYtoRPHI.vi"("X-Y"=w357) -> ("r-phi"=w359:dbl[])
              n124 = Subtract(x=w343, y=w367) -> (x-y=w360:dbl[])
              n125 = Add(x=w367, y=w343) -> (x+y=w372:dbl[])
              n126 = Index Array(array=w359, index=1) -> (element=w354:dbl)
              n127 = call "XYtoRPHI.vi"("X-Y"=w360) -> ("r-phi"=w371:dbl[])
              n128 = Divide(x=w372, y=2.0) -> (x/y=w366:dbl[])
              n129 = Index Array(array=w371, index=1) -> (element=w355:dbl)
              n130 = Subtract(x=w355, y=w354) -> (x-y=w356:dbl)
              n131 = Replace Array Subset(array=w366, new element=w356, index=3) -> (w364:dbl[])
            }
          }
        }
        "Array 2" <- w269
      }
      event "Measure Pickup Tools": Value Change {
        (unwired) "Measuring Pickup Tools" ("String")
        n132 = event-data() -> ()  [unwired: 1 in, 6 out]
        n133 = Select(t=i8 1, s=w390, f=w389) -> (s? t:f=w391:i32)
        n134 = for {
          N: w391 -> [_]
          tunnel: [w419] -> w393 mode=indexing
          tunnel: w394 -> [w423]
          tunnel: [w405] -> w392
          tunnel: w388 -> [w404] mode=indexing
          # "Default size and\norientation"
          n135 = call "Joystick and Camera SHIH VPC- external Connection.vi"("Motion in"=w423, "XYZTheta"=w404, "Measurement Point"="PickUp tool TopLeft") -> ("Motion out"=w399:refnum<class "Motion.lvclass">, "Sum"=w422:dbl[])  [unwired: 4 in, 2 out]
          n136 = Build Array(0.0 ("element"), 29.94 ("element"), 0.0 ("element"), 0.0 ("element")) -> (w410:dbl[])
          n137 = Add(x=w422, y=w410) -> (x+y=w396:dbl[])
          n138 = Array Subset(array=w396, index=0, length=2) -> (w397:dbl[])
          n139 = call-dynamic "XY Go.vi"("Speed"=20.0, "XY"=w397, "Motion in"=w399) -> ("Motion out"=w398:refnum<class "Motion.lvclass">)  [unwired: 7 in, 1 out]
          n140 = call "Joystick and Camera SHIH VPC- external Connection.vi"("Motion in"=w398, "Measurement Point"="PickUp tool BottomRight", "Inital GO"=FALSE) -> ("Motion out"=w405:refnum<class "Motion.lvclass">, "Sum"=w421:dbl[])  [unwired: 4 in, 2 out]
          n141 = Add(x=w422, y=w421) -> (x+y=w428:dbl[])
          n142 = Subtract(x=w421, y=w422) -> (x-y=w420:dbl[])
          n143 = Divide(x=w428, y=2.0) -> (x/y=w425:dbl[])
          n144 = call "XYtoRPHI.vi"("X-Y"=w420) -> ("r-phi"=w426:dbl[])
          n145 = Index Array(array=w426, index=1) -> (element=w414:dbl)
          n146 = Absolute Value(x=w414) -> (abs(x)=w417:dbl)
          n147 = Sign(1:w414) -> (0:w415:dbl)
          n148 = Subtract(x=w417, y=1.5707963267948966) -> (x-y=w416:dbl)
          n149 = Multiply(x=w415, y=w416) -> (x*y=w413:dbl)
          n150 = Replace Array Subset(array=w425, new element=w413, index=3) -> (w419:dbl[])
        }
        "Measured PickupTool position" <- w393
      }
      event "Deposit Glue": Value Change {
        # "glue box (half-width, half-length, lines)"
        # "Sensor glue pattern Sensor A then B"
        # "Unmount syringe"
        # "first needle park position\nneedle gap on Z value : 0.5 mm"
        # "Syringe-camera offset"
        n151 = event-data() -> ()  [unwired: 1 in, 6 out]
        n152 = call-poly <vilib>:"Read Delimited Spreadsheet.vi"("file path (dialog if empty)"=path "D:/INTT/V1/Assembly Data/Tool Offsets/Dispense Tip Offset.txt", "number of rows (all:-1)"=-1) -> ("first row"=w483:dbl[])  [unwired: 8 in, 5 out]
        n153 = Build Array(11.75, -22, 0.5 ("element"), 0.0 ("element")) -> (w476:dbl[])
        n154 = Index Array(array=w483, index #1=0 ("index"), index #2=1 ("index")) -> (element #1=w478:dbl, element #2=w475:dbl)
        n155 = Build Array(w478, w475, 0.0 ("element"), 0.0 ("element")) -> (w456:dbl[])
        n156 = Add(x=w456, y=w476) -> (x+y=w443:dbl[])
        n157 = Add(x=w444, y=w443) -> (x+y=w462:dbl[])
        "Needle parking position" <- w462
        n158 = call "XYZTheta Go.vi"("XYZTheta In"=w462, "Motion in"=w463) -> ("error out"=w474:errorcluster, "XYZTheta Out"=w472:dbl[], "Motion out"=w461:refnum<class "Motion.lvclass">)  [unwired: 7 in]
        n159 = call "Display Message to User"("error in (no error)"=w474) -> ("error out"=w464:errorcluster)  [unwired: 9 in, 1 out]
        n160 = Select(t=dbl[][] [[0.0, -53.0, 1.0, 4.0], [-2.81, -56.0, 4.0, 4.0], [-5.62, -59.0, 4.0, 4.0], [-8.43, -62.0, 4.0, 1.0], [0.0, -39.0, 1.0, 0.0], [-2.81, -42.0, 4.0, 0.0], [-5.62, -45.0, 4.0, 0.0], [-8.43, -48.0, 4.0, 0.0]], s=w438, f=dbl[][] [[0.0, -39.0, 1.0, 4.0], [-2.81, -42.0, 4.0, 4.0], [-5.62, -45.0, 4.0, 4.0], [-8.43, -48.0, 4.0, 1.0], [0.0, -53.0, 1.0, 0.0], [-2.81, -56.0, 4.0, 0.0], [-5.62, -59.0, 4.0, 0.0], [-8.43, -62.0, 4.0, 0.0]]) -> (s? t:f=w436:dbl[][])
        n161 = Index Array(array=w472, index=2) -> (element=w468:dbl)
        n162 = call-dynamic "Z Go.vi"("error in (no error)"=w464, "Speed"=20.0, "Position"=0.0, "Motion in"=w461) -> ("error out"=w460:errorcluster, "Motion out"=w467:refnum<class "Motion.lvclass">)  [unwired: 6 in]
        n163 = call "Display Message to User2"("error in (no error)"=w460) -> ("error out"=w459:errorcluster)  [unwired: 9 in, 1 out]
        n164 = Add(x=w468, y=-2.5) -> (x+y=w469:dbl)
        n165 = call-dynamic "Z Go.vi"("error in (no error)"=w459, "Speed"=20.0, "Position"=w469, "Motion in"=w467) -> ("error out"=w457:errorcluster, "Motion out"=w458:refnum<class "Motion.lvclass">)  [unwired: 6 in]
        n166 = call-dynamic "Connect.vi"("Ultimus V in"=refnum<class "Ultimus V2.lvclass"> refnum ("Ultimus V2.lvclass")) -> ("Ultimus V out"=w455:refnum<class "Ultimus V2.lvclass">)  [unwired: 9 in, 1 out]
        n167 = case shown="False" w447 {
          tunnel: w458 -> [w498 w611]
          tunnel: w457 -> [w499 w610]
          tunnel: [w497 w609] -> w452
          tunnel: [w499 w608] -> w450
          tunnel: w446 -> [w494 w602]
          tunnel: w456 -> [w493 w607]
          tunnel: w455 -> [w495 w606]
          tunnel: [w496 w605] -> w453
          tunnel: w445 -> [w492 w604]
          tunnel: w436 -> [w491 _]
          tunnel: "Needle Height Compenstation\n(glue gap)" -> [w490 w603]
          tunnel: "check height?" -> [w489 w600]
          frame False {
            # "two sensor, Sensor B then A"
            n168 = for {
              N: w492 -> [_]
              tunnel: w498 -> [w515]
              tunnel: [w514] -> w496
              tunnel: [w513] -> w497
              tunnel: w495 -> [w512]
              tunnel: w494 -> [w511] mode=indexing
              tunnel: w493 -> [w505]
              tunnel: w491 -> [w507]
              tunnel: w490 -> [w501]
              tunnel: w489 -> [w500]
              i -> [w503]
              # "four\nloops"
              n169 = Multiply(x=4, y=w503) -> (x*y=w502:i32)
              n170 = Array Subset(array=w507, index (row)=w502, length (row)=4 ("length"), index (col)=0, length (col)=3 ("length")) -> (w506:dbl[][])
              "GlueBox" <- w506
              n171 = for {
                N: 4 -> [_]
                tunnel: w515 -> [w578]
                tunnel: [w570] -> w514
                tunnel: [w565] -> w513
                tunnel: w512 -> [w557]
                tunnel: w511 -> [w535]
                tunnel: w506 -> [w532] mode=indexing
                tunnel: w505 -> [w538]
                tunnel: w501 -> [w524]
                tunnel: w500 -> [w521]
                n172 = Index Array(array=w532, index=0) -> (element=w554:dbl)
                n173 = Index Array(array=w532, index=1) -> (element=w553:dbl)
                n174 = Array Subset(array=w535, index=0, length=2) -> (w537:dbl[])
                n175 = Add(x=w537, y=w538) -> (x+y=w536:dbl[])
                n176 = Absolute Value(x=w554) -> (abs(x)=w552:dbl)
                n177 = Absolute Value(x=w553) -> (abs(x)=w550:dbl)
                n178 = Multiply(x=w550, y=2.0) -> (x*y=w528:dbl)
                n179 = Add(x=w536, y=w532) -> (x+y=w547:dbl[])
                n180 = Multiply(x=w552, y=2.0) -> (x*y=w529:dbl)
                n181 = Multiply(x=w528, y=-1.0) -> (x*y=w540:dbl)
                n182 = Build Array(0.0 ("element"), w528) -> (w548:dbl[])
                n183 = Build Array(w529, 0.0 ("element")) -> (w545:dbl[])
                n184 = Build Array(0.0 ("element"), w540) -> (w526:dbl[])
                n185 = Add(x=w547, y=w548) -> (x+y=w544:dbl[])
                n186 = Add(x=w544, y=w545) -> (x+y=w527:dbl[])
                n187 = call-dynamic "XY Go.vi"("Speed"=200.0, "XY"=w547, "Motion in"=w578) -> ("error out"=w530:errorcluster, "Motion out"=w577:refnum<class "Motion.lvclass">)  [unwired: 7 in]
                n188 = Add(x=w527, y=w526) -> (x+y=w525:dbl[])
                n189 = Index Array(array=w535, index=2) -> (element=w534:dbl)
                n190 = Index Array(array=w532, index=2) -> (element=w531:dbl)
                n191 = Build Array(w544, w527, w525, w547) -> (w539:dbl[][])
                "appended array" <- w539
                n192 = Add(x=w534, y=w524) -> (x+y=w563:dbl)
                n193 = call-dynamic "Z Go.vi"("error in (no error)"=w530, "Speed"=5.0, "Position"=w563, "Motion in"=w577) -> ("error out"=w523:errorcluster, "Motion out"=w573:refnum<class "Motion.lvclass">)  [unwired: 6 in]
                n194 = case shown="True" w521 {
                  tunnel: w523 -> [w591 w593]
                  tunnel: [w591 w592] -> w522
                  frame False {
                  }
                  frame True {
                    n195 = call "User11"("error in (no error)"=w593) -> ("error out"=w592:errorcluster)  [unwired: 9 in, 1 out]
                  }
                }
                n196 = call "vacuum.vi"("error in (no error)"=w522, "Vacuum Setting (0000)"=i64 100, "Ultimus V in"=w557) -> ("error out"=w575:errorcluster, "Ultimus V out"=w560:refnum<class "Ultimus V2.lvclass">)  [unwired: 7 in]
                n197 = flat-sequence {
                  tunnel: w560 -> [w584]
                  tunnel: w575 -> [w585]
                  tunnel: [w585] -> w520
                  tunnel: [w584] -> w519
                  tunnel: [w583] -> w518
                  tunnel: [w582] -> w517
                  tunnel: [w590] -> w576
                  tunnel: [w587] -> w559
                  tunnel: w520 -> [w589]
                  tunnel: w519 -> [w588]
                  tunnel: w518 -> [w586]
                  frame #0 {
                    n198 = call "air pressure setting.vi"() -> ("air pressure indecator"=w583:i32, "deposit speed 2"=w582:dbl)
                  }
                  frame #1 {
                    n199 = call-dynamic "Pressure.vi"("error in (no error)"=w589, "Pressure"=w586, "Ultimus V in"=w588) -> ("error out"=w590:errorcluster, "Ultimus V out"=w587:refnum<class "Ultimus V2.lvclass">)  [unwired: 7 in]
                  }
                }
                n200 = call-dynamic "Dispense.vi"("error in (no error)"=w576, "Ultimus V in"=w559) -> ("error out"=w572:errorcluster, "Ultimus V out"=w558:refnum<class "Ultimus V2.lvclass">)  [unwired: 8 in]
                n201 = for {
                  N: w531 -> [_]
                  tunnel: w573 -> [w599]
                  tunnel: w572 -> [w598]
                  tunnel: [w597] -> w571
                  tunnel: [w596] -> w569
                  tunnel: w539 -> [w595] mode=indexing
                  tunnel: w517 -> [_]
                  n202 = call-dynamic "XY Go.vi"("error in (no error)"=w598, "Speed"=4.5, "XY"=w595, "Motion in"=w599) -> ("error out"=w597:errorcluster, "Motion out"=w596:refnum<class "Motion.lvclass">)  [unwired: 6 in]
                }
                n203 = Add(x=w563, y=-2.0) -> (x+y=w566:dbl)
                n204 = call-dynamic "Dispense.vi"("error in (no error)"=w571, "Ultimus V in"=w558) -> ("error out"=w564:errorcluster, "Ultimus V out"=w570:refnum<class "Ultimus V2.lvclass">)  [unwired: 8 in]
                n205 = call-dynamic "Z Go.vi"("error in (no error)"=w564, "Speed"=10.0, "Position"=w566, "Motion in"=w569) -> ("Motion out"=w565:refnum<class "Motion.lvclass">)  [unwired: 6 in, 1 out]
              }
            }
          }
          frame True {
            n206 = case shown="True" w600 {
              tunnel: w602 -> [w612 w616]
              tunnel: [w612 w613] -> w601
              frame False {
              }
              frame True {
                n207 = Array Subset(array=w616, index (row)=12 ("index"), length (row)=4 ("length")) -> (w613:dbl[][])  [unwired: 2 in]
              }
            }
            n208 = for {
              N: w604 -> [_]
              tunnel: w611 -> [w656]
              tunnel: w610 -> [w655]
              tunnel: [w641] -> w605
              tunnel: [w640] -> w609
              tunnel: [w639] -> w608
              tunnel: w601 -> [w627] mode=indexing
              tunnel: w607 -> [w626]
              tunnel: w606 -> [w625]
              tunnel: w603 -> [w623]
              tunnel: w600 -> [w620]
              # "move the glue in x-dir\n0.1 mm closer to center"
              n209 = Index Array(array=w627, index=2) -> (element=w628:dbl)
              n210 = Add(x=w627, y=w626) -> (x+y=w654:dbl[])
              n211 = Build Array(0.0 ("element"), 3.3 ("element")) -> (w659:dbl[])
              n212 = Subtract(x=w654, y=w659) -> (x-y=w660:dbl[])
              n213 = Add(x=w628, y=w623) -> (x+y=w629:dbl)
              n214 = Add(x=w654, y=w659) -> (x+y=w637:dbl[])
              n215 = call-dynamic "XY Go.vi"("error in (no error)"=w655, "Speed"=200.0, "XY"=w660, "Motion in"=w656) -> ("error out"=w642:errorcluster, "Motion out"=w635:refnum<class "Motion.lvclass">)  [unwired: 6 in]
              n216 = call-dynamic "Z Go.vi"("error in (no error)"=w642, "Speed"=5.0, "Position"=w629, "Motion in"=w635) -> ("error out"=w622:errorcluster)  [unwired: 6 in, 1 out]
              n217 = case shown="True" w620 {
                tunnel: w622 -> [w669 w671]
                tunnel: [w669 w670] -> w621
                frame False {
                }
                frame True {
                  n218 = call "Display Message to User7"("error in (no error)"=w671) -> ("error out"=w670:errorcluster)  [unwired: 9 in, 1 out]
                }
              }
              n219 = call "vacuum.vi"("error in (no error)"=w621, "Vacuum Setting (0000)"=i64 100, "Ultimus V in"=w625) -> ("error out"=w651:errorcluster, "Ultimus V out"=w646:refnum<class "Ultimus V2.lvclass">)  [unwired: 7 in]
              n220 = flat-sequence {
                tunnel: w646 -> [w662]
                tunnel: w651 -> [w663]
                tunnel: [w663] -> w619
                tunnel: [w662] -> w618
                tunnel: [w661] -> w617
                tunnel: [w668] -> w652
                tunnel: [w665] -> w644
                tunnel: w619 -> [w667]
                tunnel: w618 -> [w666]
                tunnel: w617 -> [w664]
                frame #0 {
                  n221 = call "air pressure setting.vi"() -> ("air pressure indecator"=w661:i32)  [unwired: 1 out]
                }
                frame #1 {
                  n222 = call-dynamic "Pressure.vi"("error in (no error)"=w667, "Pressure"=w664, "Ultimus V in"=w666) -> ("error out"=w668:errorcluster, "Ultimus V out"=w665:refnum<class "Ultimus V2.lvclass">)  [unwired: 7 in]
                }
              }
              n223 = call-dynamic "Dispense.vi"("error in (no error)"=w652, "Ultimus V in"=w644) -> ("error out"=w636:errorcluster, "Ultimus V out"=w643:refnum<class "Ultimus V2.lvclass">)  [unwired: 8 in]
              n224 = call "Time Delay"("error in (no error)"=w636) -> ("error out"=w634:errorcluster)  [unwired: 10 in]
              n225 = call-dynamic "XY Go.vi"("error in (no error)"=w634, "Speed"=5.0, "XY"=w637, "Motion in"=w635) -> ("error out"=w633:errorcluster, "Motion out"=w631:refnum<class "Motion.lvclass">)  [unwired: 6 in]
              n226 = call "Time Delay3"("error in (no error)"=w633) -> ("error out"=w632:errorcluster)  [unwired: 10 in]
              n227 = call "Time Delay2"("error in (no error)"=w634) -> ("error out"=w645:errorcluster)  [unwired: 10 in]
              n228 = call-dynamic "Dispense.vi"("error in (no error)"=w645, "Ultimus V in"=w643) -> ("Ultimus V out"=w641:refnum<class "Ultimus V2.lvclass">)  [unwired: 8 in, 1 out]
              n229 = Add(x=w629, y=-2.5) -> (x+y=w649:dbl)
              n230 = call-dynamic "Z Go.vi"("error in (no error)"=w632, "Speed"=10.0, "Position"=w649, "Motion in"=w631) -> ("error out"=w639:errorcluster, "Motion out"=w640:refnum<class "Motion.lvclass">)  [unwired: 6 in]
            }
          }
        }
        n231 = call-dynamic "Disconnect.vi"("Ultimus V in"=w453) -> ()  [unwired: 9 in, 1 out]
        n232 = call "XYZTheta Go.vi"("error in (no error)"=w450, "XYZTheta In"=dbl[] [400.0, 625.0, 0.0, 0.1], "Motion in"=w452) -> ("error out"=w451:errorcluster, "Motion out"=w448:refnum<class "Motion.lvclass">)  [unwired: 6 in, 1 out]
        n233 = call "Display Message to User3"("error in (no error)"=w451) -> ()  [unwired: 9 in, 2 out]
      }
      event "Needle Alignment": Value Change {
        (unwired) "Needle Alignment in progress ...." ("String")
        # "first needle park position\nneedle gap on Z value : 0.5 mm"
        # "Syringe-camera offset"
        n234 = event-data() -> ()  [unwired: 1 in, 6 out]
        n235 = call-poly <vilib>:"Read Delimited Spreadsheet.vi"("file path (dialog if empty)"=path "D:/INTT/V1/Assembly Data/Tool Offsets/Dispense Tip Offset.txt", "number of rows (all:-1)"=-1) -> ("first row"=w714:dbl[])  [unwired: 8 in, 5 out]
        n236 = Build Array(11.75, -22, 0.5 ("element"), 0.0 ("element")) -> (w707:dbl[])
        n237 = Index Array(array=w714, index #1=0 ("index"), index #2=1 ("index")) -> (element #1=w709:dbl, element #2=w706:dbl)
        n238 = Build Array(w709, w706, 0.0 ("element"), 0.0 ("element")) -> (w676:dbl[])
        n239 = Add(x=w676, y=w707) -> (x+y=w700:dbl[])
        n240 = Add(x=w699, y=w700) -> (x+y=w701:dbl[])
        n241 = call "XYZTheta Go.vi"("XYZTheta In"=w701, "Motion in"=w691) -> ("error out"=w705:errorcluster, "XYZTheta Out"=w681:dbl[], "Motion out"=w690:refnum<class "Motion.lvclass">)  [unwired: 7 in]
        n242 = call "Display Message to User10"("error in (no error)"=w705) -> ("error out"=w702:errorcluster)  [unwired: 9 in, 1 out]
        n243 = call-dynamic "Z Go.vi"("error in (no error)"=w702, "Speed"=20.0, "Position"=0.0, "Motion in"=w690) -> ("Motion out"=w689:refnum<class "Motion.lvclass">)  [unwired: 6 in, 1 out]
        n244 = Replace Array Subset(array=w681, new element=0.0 ("new element/subarray"), index=2) -> (w678:dbl[])
        n245 = call "Joystick and Camera SHIH VPC- external Connection.vi"("Motion in"=w689, "XYZTheta"=w678, "Measurement Point"="Touch Needle on a surface") -> ("Motion out"=w687:refnum<class "Motion.lvclass">, "Gantry"=w677:dbl[])  [unwired: 4 in, 2 out]
        n246 = Subtract(x=w677, y=w676) -> (x-y=w675:dbl[])
        n247 = call "Joystick and Camera SHIH VPC- external Connection.vi"("Motion in"=w687, "XYZTheta"=w675, "Measurement Point"="Measure the touch spot with camera") -> ("Motion out"=w683:refnum<class "Motion.lvclass">, "Gantry"=w686:dbl[])  [unwired: 4 in, 2 out]
        n248 = Subtract(x=w677, y=w686) -> (x-y=w685:dbl[])
        n249 = call-poly <vilib>:"Write Delimited Spreadsheet.vi"("file path (dialog if empty)"=path "D:/INTT/V1/Assembly Data/Tool Offsets/Dispense Tip Offset.txt", "1D data"=w685, "append to file? (new file:F)"=FALSE) -> ()  [unwired: 11 in, 2 out]
      }
      event "Pick and place": Value Change {
        (unwired) "PICK and PLACE samples ..." ("String")
        (unwired) -21.3804 ("new element/subarray")
        n250 = event-data() -> ()  [unwired: 1 in, 6 out]
        n251 = call-poly <vilib>:"Read Delimited Spreadsheet.vi"("file path (dialog if empty)"=path "D:/INTT/V1/Assembly Data/Tool Offsets/Bellows Tool Offset.txt", "number of rows (all:-1)"=-1) -> ("first row"=w745:dbl[])  [unwired: 8 in, 5 out]
        n252 = Select(t=1, s=w722, f=w734) -> (s? t:f=w750:i32)
        n253 = Index Array(array=w745, index #1=0 ("index"), index #2=1 ("index"), index #3=2 ("index")) -> (element #1=w741:dbl, element #2=w740:dbl, element #3=w739:dbl)
        n254 = case shown="True" w730 {
          tunnel: [w751 w754] -> w729
          tunnel: w724 -> [w751 w753]
          frame False {
          }
          frame True {
            # "sensor A"
            # "sensor B"
            n255 = Index Array(array=w753, index=0) -> (element=w752:i32)
            n256 = Index Array(array=w753, index=1) -> (element=w755:i32)
            n257 = Build Array(w755, w752) -> (w754:i32[])
          }
        }
        n258 = for {
          N: w750 -> [_]
          tunnel: w734 -> [w794]
          tunnel: w735 -> [w790]
          tunnel: w748 -> [w814]
          tunnel: [w802] -> w738
          tunnel: w736 -> [w812] mode=indexing
          tunnel: [w778] -> w728
          tunnel: w727 -> [w766]
          tunnel: w741 -> [w804]
          tunnel: w740 -> [w803]
          tunnel: w737 -> [w787]
          tunnel: w739 -> [w801]
          tunnel: w722 -> [w771]
          tunnel: w729 -> [w760] mode=indexing
          tunnel: "VacChannel for sample" -> [w773]
          tunnel: "check height? 2" -> [w758]
          tunnel: w722 -> [w759]
          i -> [w780]
          w764 = 0 ("Channel")
          w763 = TRUE ("Value")
          # "put back pickup tool"
          # "if chips, do one pickup tool and multiple samples;\nif sensors, one pickup tool for one sample ( so 2->2);"
          # "build a fake 2d arrays"
          # "sensor"
          # "chip pickup tool"
          # "pickup tool height offset"
          # "Pick up PICKUP TOOL"
          # "Pick up CHIPs/Sensor and place on HDI"
          n259 = Select(t=w794, s=w771, f=1) -> (s? t:f=w793:i32)
          n260 = Build Array(w804, w803, w801, 0.0 ("element")) -> (w799:dbl[])
          n261 = Add(x=w812, y=w799) -> (x+y=w800:dbl[])
          n262 = call "XYZTheta-2Zspeed Go.vi"("XYZTheta In"=w800, "Motion in"=w814) -> ("error out"=w762:errorcluster, "Motion out"=w813:refnum<class "Motion.lvclass">)  [unwired: 7 in, 1 out]
          n263 = Select(t=-18.52 ("new element/subarray"), s=w771, f=-13.13 ("t")) -> (s? t:f=w795:dbl)
          n264 = call "WriteReadWait.vi"("Read Value"=w763, "Write Value"=w763, "error in (no error)"=w762, "Read"=w764, "Write"=w764, "I-O in"=w766) -> ("error out"=w761:errorcluster, "I-O out"=w765:refnum<class "NI-DAQ.lvclass">)  [unwired: 4 in]
          n265 = Replace Array Subset(array=w799, new element=w795, index=2) -> (w797:dbl[])
          n266 = Index Array(array=w790, index (row)=w780) -> (element=w789:dbl[])  [unwired: 1 in]
          n267 = call "Time Delay8"("error in (no error)"=w761) -> ("error out"=w810:errorcluster)  [unwired: 10 in]
          n268 = Build Array(w789, w789) -> (w788:dbl[][])
          n269 = Select(t=w790, s=w771, f=w788) -> (s? t:f=w791:dbl[][])
          n270 = Index Array(array=w787, index (row)=w780) -> (element=w786:dbl[])  [unwired: 1 in]
          n271 = Build Array(w786, w786) -> (w785:dbl[][])
          n272 = Select(t=w787, s=w771, f=w785) -> (s? t:f=w768:dbl[][])
          n273 = case shown="False" w758 {
            tunnel: [w815 w817] -> w767
            tunnel: w768 -> [w815 w816]
            frame False {
            }
            frame True {
              n274 = Array Subset(array=w816, index (row)=12 ("index"), length (row)=4 ("length")) -> (w817:dbl[][])  [unwired: 2 in]
            }
          }
          n275 = Select(t="chip placement height compensation", s=w771, f=0.0) -> (s? t:f=w769:dbl)
          n276 = for {
            N: w793 -> [_]
            tunnel: w791 -> [w834] mode=indexing
            tunnel: w813 -> [w836]
            tunnel: w797 -> [w835]
            tunnel: w810 -> [w833]
            tunnel: [w832] -> w805
            tunnel: w765 -> [w831]
            tunnel: w767 -> [w828] mode=indexing
            tunnel: [w827] -> w796
            tunnel: w769 -> [w826]
            tunnel: w760 -> [w825]
            tunnel: w773 -> [w824]
            tunnel: [w823] -> w772
            tunnel: w771 -> [w822]
            tunnel: w758 -> [w821]
            tunnel: w759 -> [w820]
            n277 = flat-sequence {
              tunnel: w834 -> [w853]
              tunnel: [w855] -> w837
              tunnel: w836 -> [w854]
              tunnel: w835 -> [w852]
              tunnel: w833 -> [w850]
              tunnel: w831 -> [w848]
              tunnel: [w842] -> w830
              tunnel: [w843] -> w829
              tunnel: w825 -> [w845]
              tunnel: w824 -> [w840]
              tunnel: w837 -> [w881]
              tunnel: [w880] -> w832
              tunnel: w835 -> [w878]
              tunnel: w830 -> [w879]
              tunnel: w829 -> [w866]
              tunnel: w828 -> [w877]
              tunnel: [w856] -> w827
              tunnel: w826 -> [w870]
              tunnel: w824 -> [w865]
              tunnel: [w861] -> w823
              tunnel: w822 -> [_]
              tunnel: w821 -> [w867]
              tunnel: w820 -> [w860]
              frame #0 {
                w841 = TRUE ("Value")
                w844 = FALSE ("Value")
                # "pickup sample"
                # "release sample from tray"
                # "pickup sample from tray"
                n278 = Add(x=w853, y=w852) -> (x+y=w851:dbl[])
                n279 = call "XYZTheta-2Zspeed Go.vi"("error in (no error)"=w850, "XYZTheta In"=w851, "Motion in"=w854) -> ("error out"=w849:errorcluster, "Motion out"=w855:refnum<class "Motion.lvclass">)  [unwired: 6 in, 1 out]
                n280 = call "Time Delay4"("error in (no error)"=w849) -> ("error out"=w846:errorcluster)  [unwired: 10 in]
                n281 = call "WriteReadWait.vi"("Read Value"=w844, "Write Value"=w844, "error in (no error)"=w846, "Read"=w845, "Write"=w845, "I-O in"=w848) -> ("error out"=w847:errorcluster, "I-O out"=w839:refnum<class "NI-DAQ.lvclass">)  [unwired: 4 in]
                n282 = call "Time Delay11"("error in (no error)"=w847) -> ("error out"=w838:errorcluster)  [unwired: 10 in]
                n283 = call "WriteReadWait.vi"("Read Value"=w841, "Write Value"=w841, "error in (no error)"=w838, "Read"=w840, "Write"=w840, "I-O in"=w839) -> ("error out"=w842:errorcluster, "I-O out"=w843:refnum<class "NI-DAQ.lvclass">)  [unwired: 4 in]
              }
              frame #1 {
                w863 = FALSE ("Value")
                # "release sample on HDI"
                # "lift for chip/sensor thickness"
                # "place sample on HDI"
                n284 = Add(x=w877, y=w878) -> (x+y=w873:dbl[])
                n285 = Build Array(0.0 ("element"), 0.0 ("element"), w870, 0.0 ("element")) -> (w872:dbl[])
                n286 = Add(x=w873, y=w872) -> (x+y=w871:dbl[])
                n287 = call "XYZTheta-2Zspeed Go.vi"("error in (no error)"=w879, "XYZTheta In"=w871, "Motion in"=w881) -> ("error out"=w869:errorcluster, "Motion out"=w880:refnum<class "Motion.lvclass">)  [unwired: 6 in, 1 out]
                n288 = case shown="False" w867 {
                  tunnel: w869 -> [w887 w889]
                  tunnel: [w887 w888] -> w868
                  frame False {
                  }
                  frame True {
                    n289 = call "Display Message to User6"("error in (no error)"=w889) -> ("error out"=w888:errorcluster)  [unwired: 9 in, 1 out]
                  }
                }
                n290 = case shown="False" w860 {
                  tunnel: w868 -> [w884 w886]
                  tunnel: [w882 w885] -> w864
                  frame False {
                    n291 = call "Time Delay7"("error in (no error)"=w884) -> ("error out"=w883:errorcluster)  [unwired: 10 in]
                    n292 = call "ser8"("error in (no error)"=w883) -> ("error out"=w882:errorcluster)  [unwired: 9 in, 1 out]
                  }
                  frame True {
                    n293 = call "Time Delay6"("error in (no error)"=w886) -> ("error out"=w885:errorcluster)  [unwired: 10 in]
                  }
                }
                n294 = call "WriteReadWait.vi"("Read Value"=w863, "Write Value"=w863, "error in (no error)"=w864, "Read"=w865, "Write"=w865, "I-O in"=w866) -> ("error out"=w862:errorcluster, "I-O out"=w861:refnum<class "NI-DAQ.lvclass">)  [unwired: 4 in]
                n295 = call "Time Delay5"("error in (no error)"=w862) -> ("error out"=w859:errorcluster)  [unwired: 10 in]
                n296 = call "message 10"("error in (no error)"=w859) -> ("error out"=w858:errorcluster)  [unwired: 9 in, 1 out]
                n297 = call "Time Delay12"("error in (no error)"=w858) -> ("error out"=w857:errorcluster)  [unwired: 10 in]
                n298 = call "message 9"("error in (no error)"=w857) -> ("error out"=w856:errorcluster)  [unwired: 9 in, 1 out]
              }
            }
          }
          n299 = call "XYZTheta-2Zspeed Go.vi"("error in (no error)"=w796, "XYZTheta In"=w800, "Motion in"=w805) -> ("error out"=w770:errorcluster, "Motion out"=w809:refnum<class "Motion.lvclass">)  [unwired: 6 in, 1 out]
          n300 = call "Time Delay9"("error in (no error)"=w770) -> ("error out"=w776:errorcluster)  [unwired: 10 in]
          n301 = call-dynamic "Digital Write 1 Channel.vi"("DAQ Module"=0, "error constant"=w776, "Value"=FALSE, "Channel"=0, "NI-DAQ.lvclass"=w772) -> ("error IO"=w779:errorcluster, "NI-DAQ.lvclass 2"=w778:refnum<class "NI-DAQ.lvclass">)  [unwired: 5 in]
          n302 = call "Time Delay10"("error in (no error)"=w779) -> ("error out"=w806:errorcluster)  [unwired: 10 in]
          n303 = call-dynamic "Z Go.vi"("error in (no error)"=w806, "Speed"=20.0, "Position"=0.0 ("new element/subarray"), "Motion in"=w809) -> ("Motion out"=w802:refnum<class "Motion.lvclass">)  [unwired: 6 in, 1 out]
        }
      }
      event "GOTO": Value Change {
        (unwired) "GOING to a position" ("String")
        n304 = event-data() -> ()  [unwired: 1 in, 6 out]
        n305 = call "XYZTheta-2Zspeed Go.vi"("XYZTheta In"="Parking position", "Motion in"=w894) -> ("Motion out"=w893:refnum<class "Motion.lvclass">)  [unwired: 7 in, 2 out]
      }
      event "READ Position": Value Change {
        n306 = event-data() -> ()  [unwired: 1 in, 6 out]
        n307 = call-dynamic "Get Current Position.vi"("Motion in"=w917) -> ("XYZTheta Out"=→"Gantry current position":dbl[], "Motion out"=w916:refnum<class "Motion.lvclass">)  [unwired: 8 in, 1 out]
      }
      event "TrayVaccum": Value Change {
        n308 = event-data() -> ()  [unwired: 1 in, 6 out]
        n309 = Index Array(array=w921, index=0) -> (element=w930:i32)
        n310 = Index Array(array="Values", index=0) -> (element=w924:bool)
        n311 = call "WriteReadWait.vi"("Read Value"=w924, "Write Value"=w924, "Read"=w930, "Write"=w930, "I-O in"=w933) -> ("error out"=w929:errorcluster, "I-O out"=w932:refnum<class "NI-DAQ.lvclass">)  [unwired: 5 in]
        n312 = Index Array(array=w921, index=1) -> (element=w927:i32)
        n313 = Index Array(array="Values", index=1) -> (element=w922:bool)
        n314 = call "WriteReadWait.vi"("Read Value"=w922, "Write Value"=w922, "error in (no error)"=w929, "Read"=w927, "Write"=w927, "I-O in"=w932) -> ("I-O out"=w919:refnum<class "NI-DAQ.lvclass">)  [unwired: 4 in, 1 out]
      }
      event Timeout {
        n315 = event-data() -> ()  [unwired: 1 in, 3 out]
        n316 = call-dynamic "Digital Read Multiple Channels.vi"("Array"=w948, "NI-DAQ in"=w947) -> ("subarray"=w949:bool[], "NI-DAQ out"=w945:refnum<class "NI-DAQ.lvclass">)  [unwired: 7 in, 1 out]
      }
    }
    "Measure HDI top-left" <- w42
    "Sample on HDI" <- w14
    "vacuum on?" <- w18
    "Sample on HDI aspect to drawing" <- w13
    n317 = feedback-in #1(w40) -> ()
    n318 = feedback-in #2(w42) -> ()
    n319 = feedback-in #3(w37) -> ()
    n320 = feedback-in #4(w29) -> ()
    n321 = feedback-in #5(w26) -> ()
    n322 = feedback-in #6(w18) -> ()
    n323 = feedback-in #7(w34) -> ()
    n324 = feedback-in #9(w13) -> ()
    n325 = feedback-in #10(w35) -> ()
    "# of tasks excuted" <- w31
  }
  n326 = call-dynamic "Disconnect.vi"("I-O in"=w1) -> ()  [unwired: 9 in, 1 out]
  n327 = call-dynamic "Disconnect.vi"("Controller in"=w4) -> ()  [unwired: 9 in, 1 out]
